vi "4Pi Capture Manager.vi"(7 "Calling VI Ref":refnum<vi>) -> ()   [LabVIEW 2016]
uses:
  4Pi Capture Manager Controls/4Pi Capture Switch Laser.ctl
  4Pi Capture Manager Controls/4Pi Capture Switch Line Scan Modes.ctl
  4Pi Capture Manager Controls/4Pi Capture Line Scan Settings.ctl
  <vilib>/Utility/miscctls.llb/LVPointTypeDef.ctl
  4Pi Capture Manager Controls/4Pi Capture Notifier Type.ctl
  4Pi Capture Manager Controls/4Pi Capture Actions.ctl
  <vilib>/vision/Image Controls.llb/IMAQ Image.ctl
  Hardware Configuration/Hardware Configuration Controls/Device Type.ctl
  Hardware Configuration/Hardware Configuration Controls/Device Function.ctl
  Device Library/Cameras/Hamamatsu/Orca Flash/Orca Flash Controls/Orca Flash Actions.ctl
  Device Library/Cameras/Hamamatsu/Orca Flash/Orca Flash Controls/Orca Flash Parameters.ctl
  Device Library/Cameras/Hamamatsu/Orca Flash/Orca Flash Controls/Orca Flash Parameter List.ctl
  Device Library/Cameras/Hamamatsu/Orca Flash/Orca Flash Controls/Orca Flash ROI.ctl
  4Pi Capture Manager Controls/4Pi Capture Scan Tracker.ctl
  Device Manager/Common Device Queue/Common Device Controls/Common Device Actions.ctl
  Device Library/DAQmx/AO Single Channel Triggered Ramp/AO SCTR Type Defs/AO SCTR Actions.ctl
  Wide Field Drift Correction/WFDC Controls/WFDC External Sync.ctl
  Wide Field Drift Correction/WFDC Controls/WFDC Cycle Pause.ctl
  Wide Field Drift Correction/WFDC Controls/WFDC Status.ctl
  Device Library/Stages/Stages Controls/Stage Actions.ctl
  Device Library/Shutters/Shutter Controls/Shutter Actions.ctl
  Device Library/AOTF and AOM/AOTF Controls/AOTF Actions.ctl
  Device Library/Cameras/Camera Controls/Camera IMAQ Key Info.ctl
  <vilib>/Utility/file.llb/Read Delimited Spreadsheet (DBL).vi
  shell32.dll
panel:
  in  "Main Tab":T1(tab)
  out "Frame":u32(slide) scale=0.0..2.0
  out "Cycle":sgl(slide) scale=0.0..1.0
  in  "Base Save Path":path
  in  "Capture":bool
  in  "Live Preview":bool
  in  "Auto Shutter":bool=TRUE
  out "Z Step":sgl(slide) scale=0.0..1.0
  in  "File Name":string="Test Image"
  in  "Preview Exposure Time (s)":dbl=0.1 caption="Exposure Time (s)"
  in  "Capture Exposure Time (s)":dbl=0.1 caption="Exposure Time (s)"
  in  "No. of Frames":u32=1 min=1
  in  "No. of Cycles":u16=1 min=1
  in  "No. of Z Steps":u16=1 min=1
  in  "Z Step Size (µm)":dbl min=-10.0 max=10.0
  in  "Switch Laser At":T2=enum."Each Cycle"
  out "Current Cycle":u16
  out "Current Step":u16
  out "Current Frame":u32
  in  "Auto Update Subfolder":bool=TRUE
  in  "Subfolder Name":string="Area"
  in  "Current Laser":u16(ring) items=["560", "642"]
  in  "Save As Preset":bool
  in  "Line Scan Active":bool
  in  "Number of Lines":u32=8 min=1 max=200 step=1
  in  "Line Scan Mode":T3
  in  "Line Scanning Presets":u16(ring) items=["01 FPS", "02 FPS", "04 FPS", "08 FPS", "16 FPS", "40 FPS"]
  in  "Line Scan Settings":T4
  in  "Camera Settings":bool
  in  "Quadrants On/Off":bool
  in  "Quit":bool
  # "Live Preview"
  # "Capture"
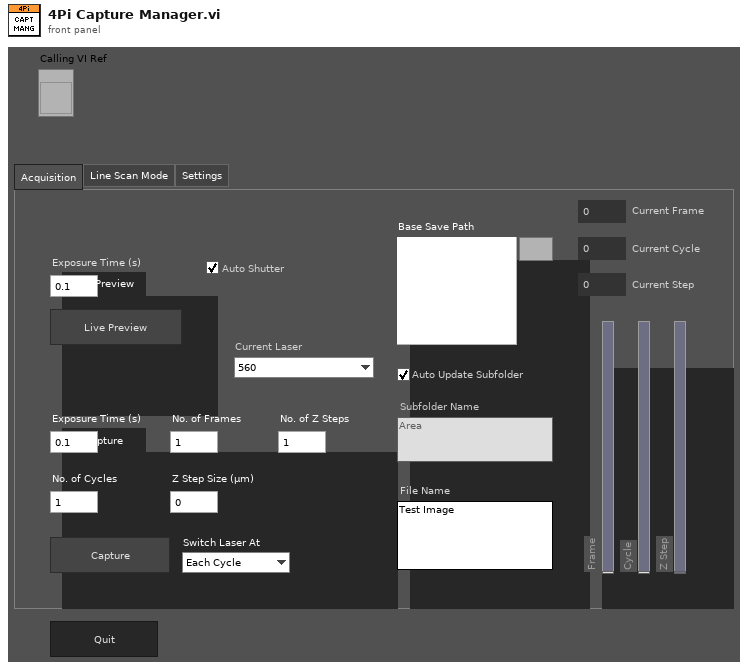
[diagram p1: front panel]
types:
  T1 = enum32{"Acquisition", "Line Scan Mode", "Settings"}
  T2 = typedef "4Pi Capture Switch Laser.ctl" = enum16{"Each Step", "Each Cycle", "All Cycles"}
  T3 = typedef "4Pi Capture Switch Line Scan Modes.ctl" = enum32{"Automatic", "Use Presets", "Manual"}
  T4 = typedef "4Pi Capture Line Scan Settings.ctl" = cluster{"Interline Interval":dbl, "Offset (V)":dbl, "Amplitude (V)":dbl, "Samples Per Channel":dbl, "Delay (ms)":dbl}
  T5 = typedef "IMAQ Image.ctl" = refnum<image>
  T6 = cluster{"Image Ref":T5, "Cycle Number":u16, "Camera Running?":bool, "Capture?":bool}
  T7 = enum8{"Enabled", "Disabled", "Disabled and Grayed Out"}
  T8 = typedef "Device Type.ctl" = enum16{"AOTF", "Camera", "Deformable Mirror", "Laser", "Shutter", "Stage", "Waveform", "Email"}
  T9 = typedef "4Pi Capture Notifier Type.ctl" = cluster{"Actions":T10, "Running?":bool, "Preview Exposure (s)":dbl, "Capture Exposure (s)":dbl, "Cycles":u16, "Frames":u32, "No. of Z Steps":u16, "Z Step Size (µm)":dbl, "Base Path":path, "Init Z Position (µm)":dbl, "Lasers Lines":string[], "Save Path":path, "Line Scan?":bool, "Line Scan Mode":T3, "Metadata File Ref":refnum<file>}
  T10 = typedef "4Pi Capture Actions.ctl" = enum16{"Idle", "Live Preview", "Capture", "Laser On", "Laser Off", "Open Shutters", "Close Shutters", "Set Exposure Time", "Start Acquisition", "Update SubFolder", "Setup", "Camera", "Switch", "Step", "Cycle", "External Cycle Sync", "Write Metadata", "Abort", "Quit"}
  T11 = enum16{"Always On", "Always Off", "Off While Running"}
  T12 = typedef "LVPointTypeDef.ctl" = cluster{"Horizontal":i16, "Vertical":i16}
  T13 = typedef "Image Type" = u32
  T14 = enum32{"Page Enabled", "Page Disabled", "Page Disabled & Grayed"}
  T15 = typedef "Device Function.ctl" = enum16{"Primary", "Secondary", "Overview", "Wide Field Drift Correction", "642 nm Excitation", "560 nm Excitation", "546 nm Excitation", "488 nm Excitation", "405 nm Excitation", "Objective Drift Correction", "4Pi Objective Lock", "Objective XY", "Objective Z", "Sample XY", "Sample Coarse Z", "Sample Z", "4Pi Lower", "4Pi Upper", "Adj Cavity", "Line Scanning", "Alert"}
  T16 = typedef "Orca Flash ROI.ctl" = cluster{"H Offset":i32, "V Offset":i32, "H Width":i32, "V Width":i32}
  T17 = typedef "Orca Flash Parameters.ctl" = cluster{"Value":dbl, "Parameter":T18}
  T18 = typedef "Orca Flash Parameter List.ctl" = u32
  T19 = typedef "Orca Flash Actions.ctl" = enum16{"IDLE", "PREVIEW", "RECORD", "Record Settings", "SETPARAM", "GETPARAM", "SETROI", "GETROI", "PROGRESSIVE MODE", "AREA MODE", "STATUS", "QUIT"}
  T20 = typedef "4Pi Capture Scan Tracker.ctl" = cluster{"Current Step":u16, "Current Cycle":u16, "Current Laser":u16, "# of Lasers":u16, "# of Cycles":u16, "# of Steps":u16, "Switch Laser At":T2}
  T21 = typedef "WFDC Status.ctl" = enum16{"Idle", "Busy", "DC Active", "Error"}
  T22 = typedef "WFDC External Sync.ctl" = cluster{"Cycle Sync":T23, "Z Offset":dbl, "WFDC Status":T21}
  T23 = typedef "WFDC Cycle Pause.ctl" = enum16{"Pause Requested", "Paused", "Resume Requested", "Resumed"}
  T24 = typedef "Stage Actions.ctl" = enum16{"Get Position", "MVR", "MOVE", "HALT", "ONTARGET", "ERROR", "REFERENCE", "INIT", "VELOCITY", "STATUS", "EXIT", "HOME", "ZEROPOS", "NANOPOS", "ANALOG", "QUIT"}
  T25 = typedef "Shutter Actions.ctl" = enum16{"Open", "Close", "Toggle", "Status", "Quit"}
  T26 = typedef "AOTF Actions.ctl" = enum16{"Error Check", "Blank", "Line On/Off", "Set Power", "Status", "Quit"}
  T27 = typedef "AO SCTR Actions.ctl" = enum16{"Stop at Offset", "Update and Run", "Quit"}
  T28 = enum16{"open", "replace", "create", "open or create", "replace or create", "replace or create with confirmation"}
  T29 = typedef "Camera IMAQ Key Info.ctl" = cluster{"Frame":u32, "Sensor Height":i32, "Sensor Width":i32, "ROI Height":i32, "ROI Width":i32, "ROI Enable?":bool, "Bit per Pixel":u8}
  T30 = typedef "Common Device Actions.ctl" = enum16{"Specific Action", "Open Front Panel", "Close Front Panel", "Quit", "Quit All"}
  T31 = typedef "LVRectTypeDef.ctl" = cluster{"Left":i16, "Top":i16, "Right":i16, "Bottom":i16}
  T32 = typedef "LVBoundsTypeDef.ctl" = cluster{"Width":u32, "Height":u32}
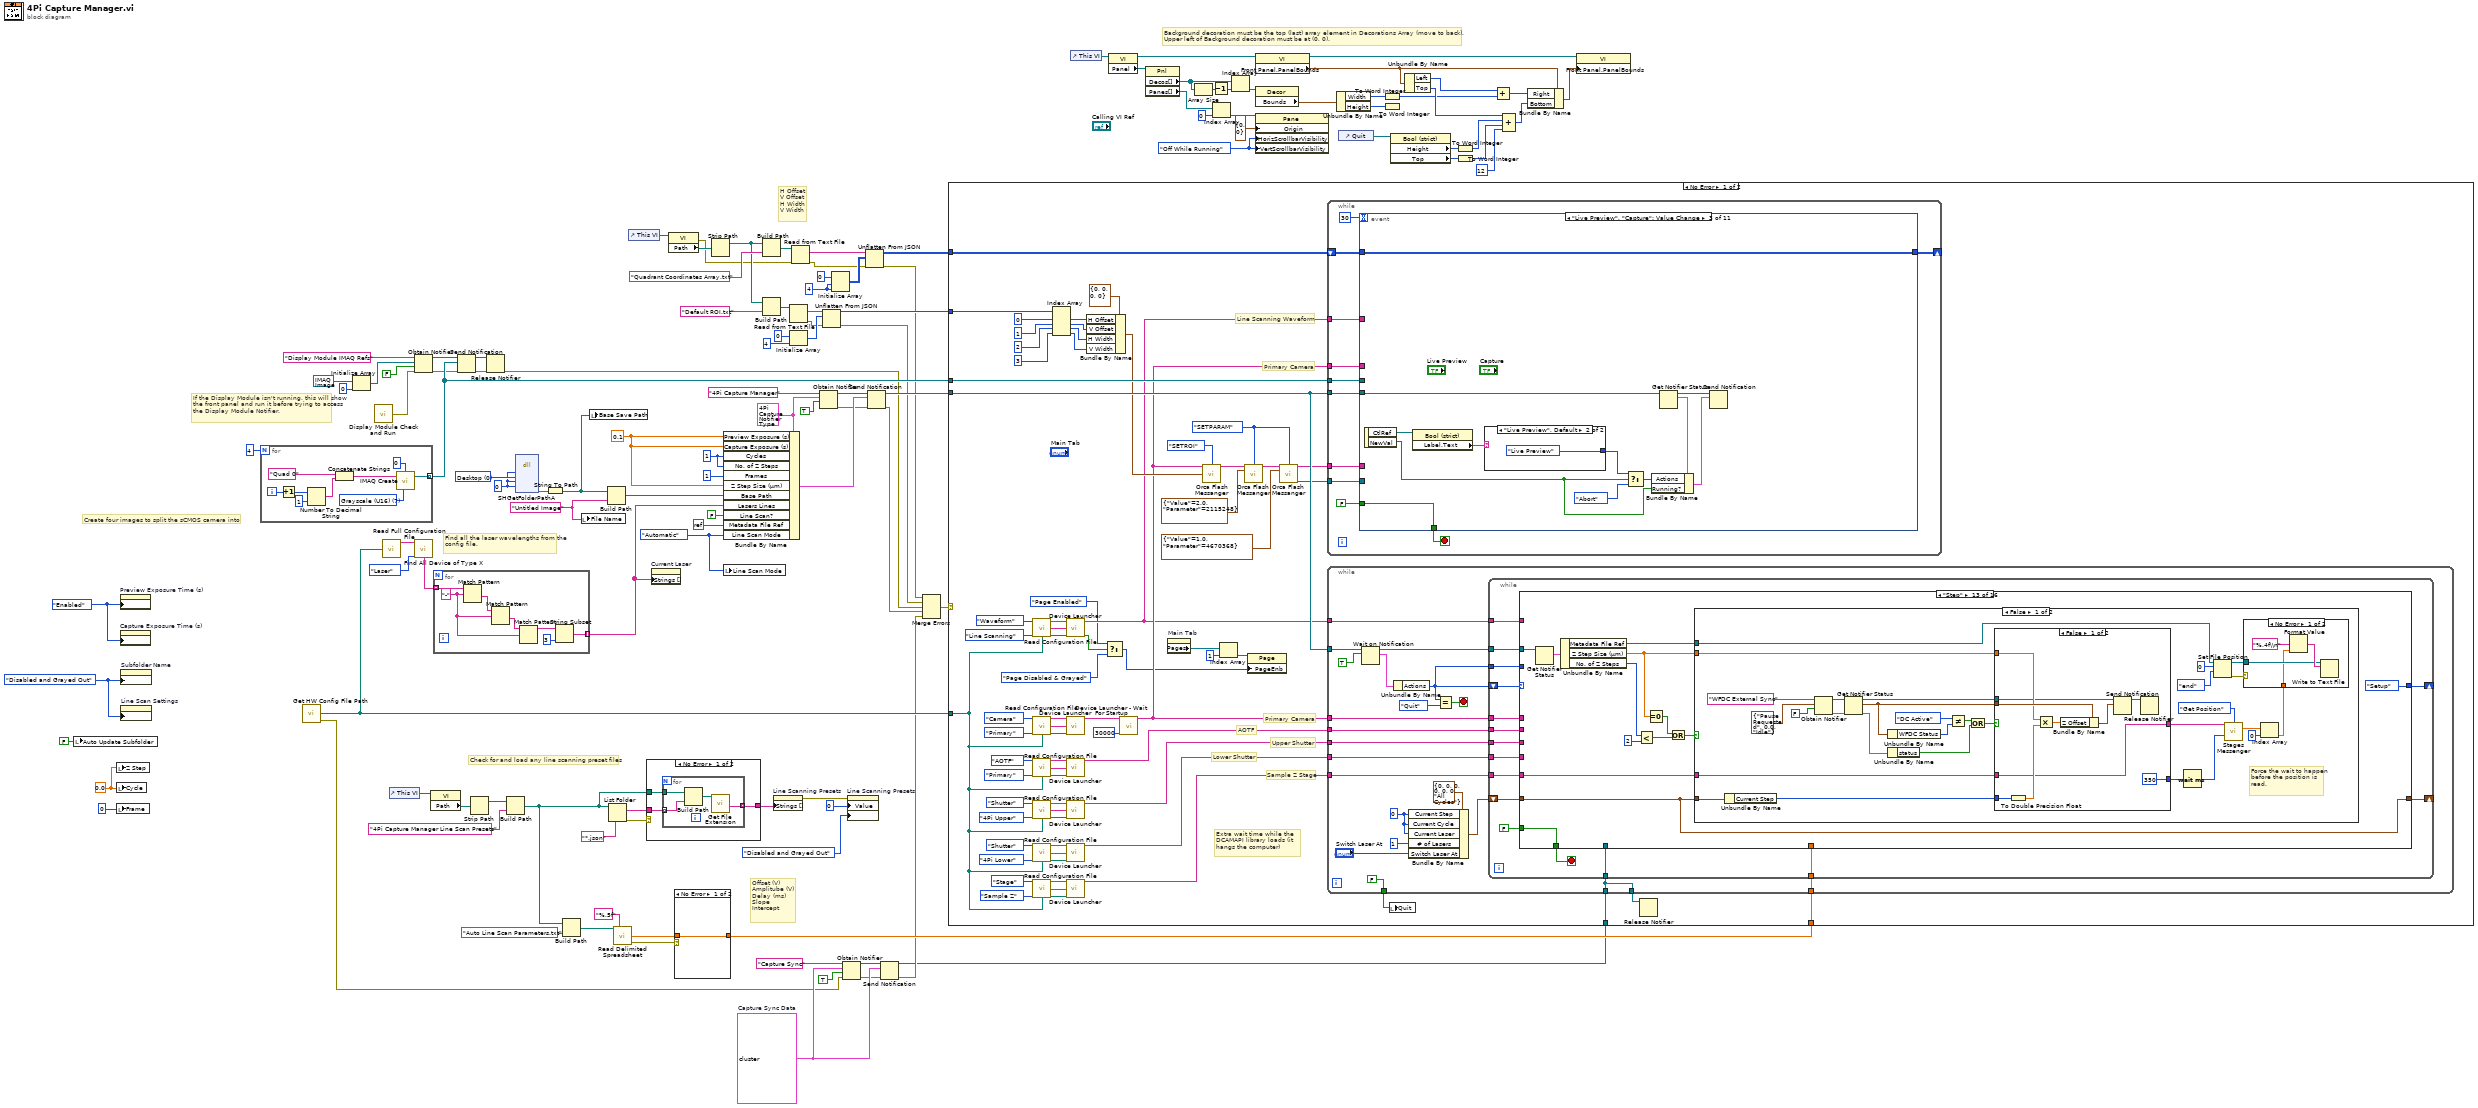
[diagram p0: block diagram]
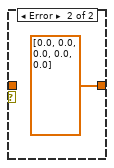
[diagram p2: hidden frame]
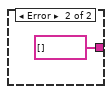
[diagram p3: hidden frame]
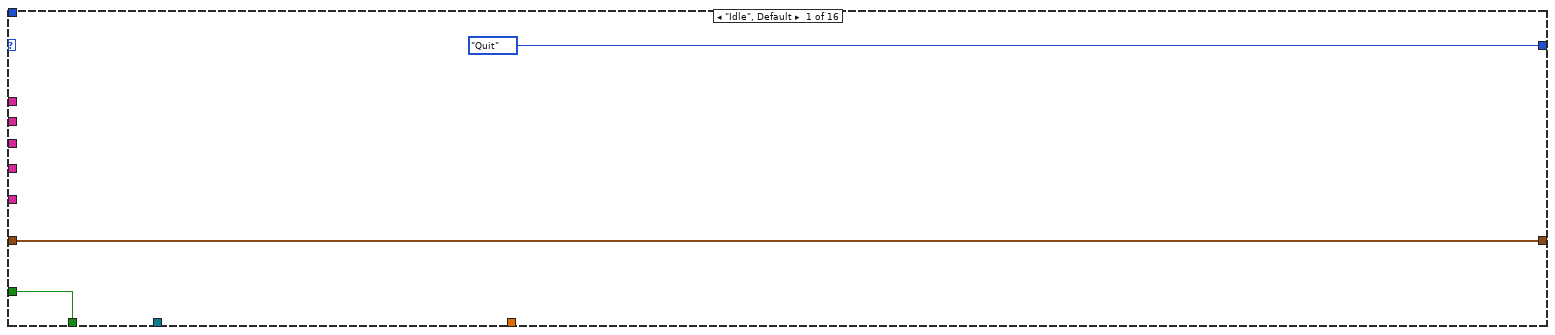
[diagram p4: hidden frame]
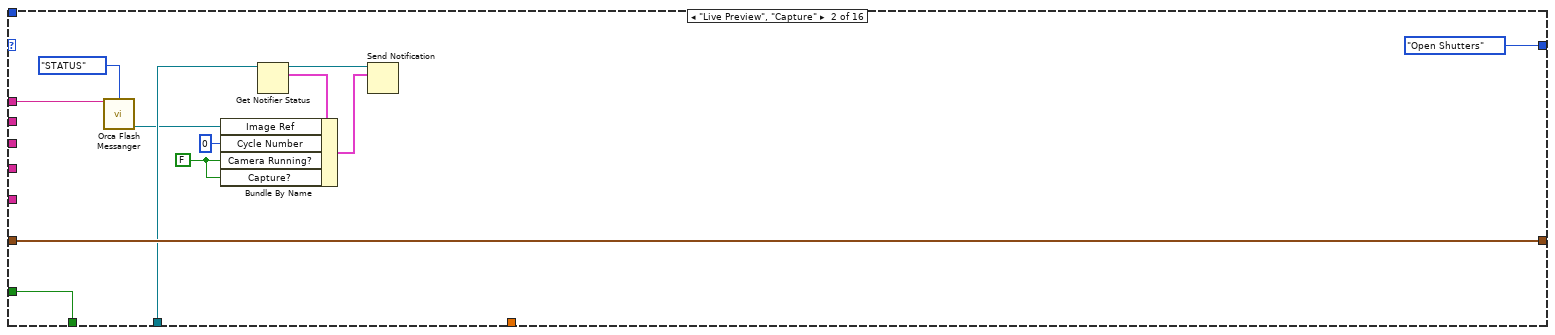
[diagram p5: hidden frame]
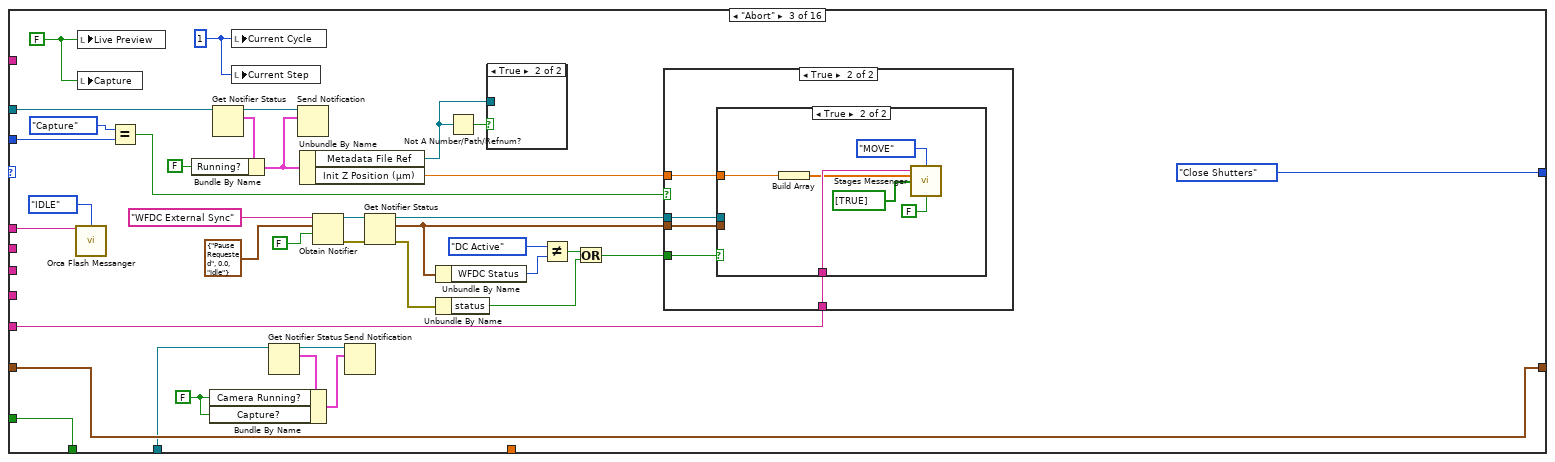
[diagram p6: hidden frame]
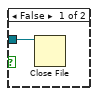
[diagram p7: hidden frame]
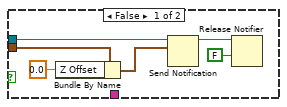
[diagram p9: hidden frame]
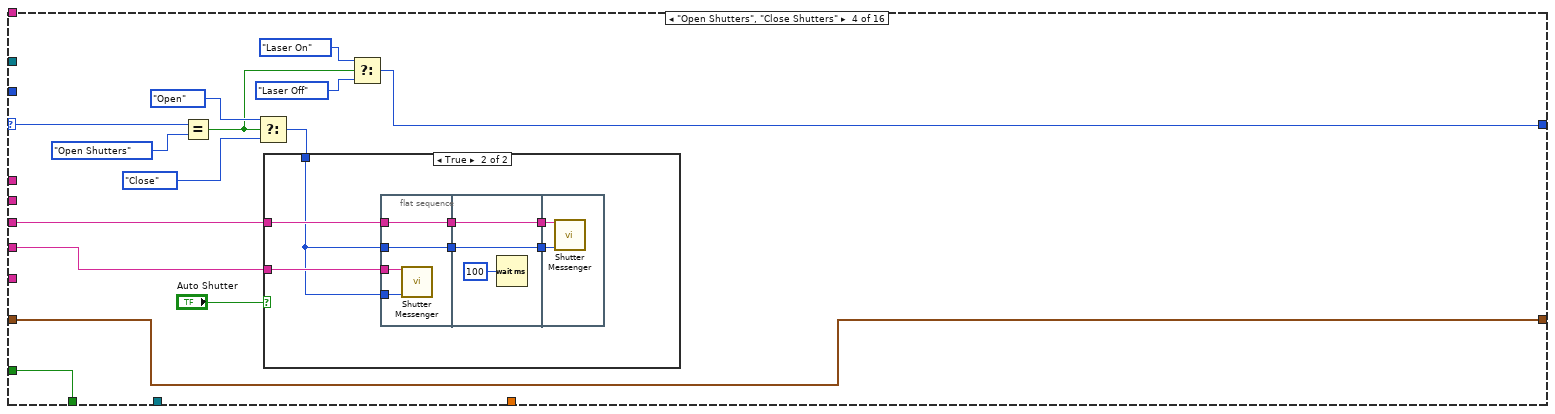
[diagram p10: hidden frame]
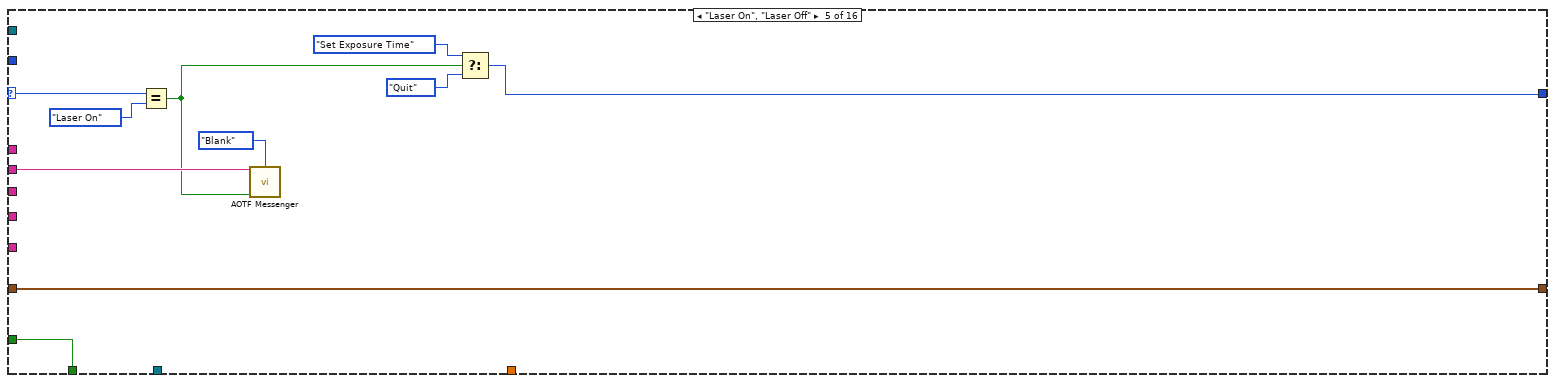
[diagram p12: hidden frame]
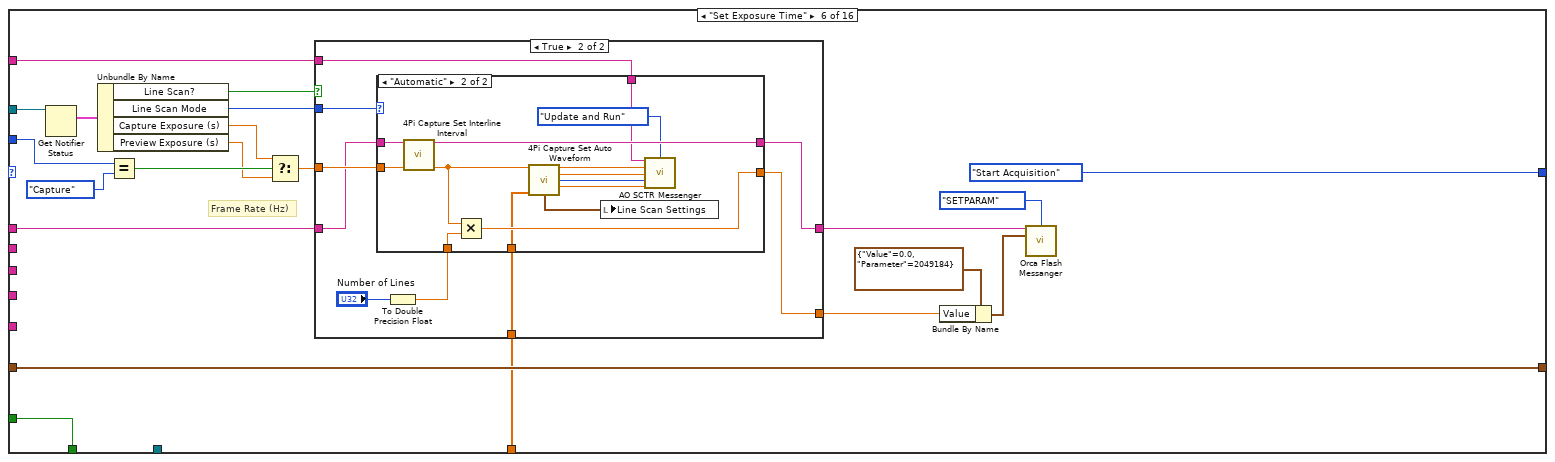
[diagram p13: hidden frame]
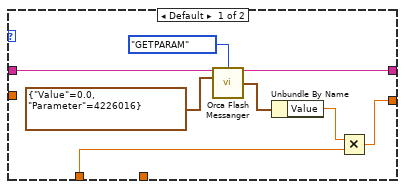
[diagram p15: hidden frame]
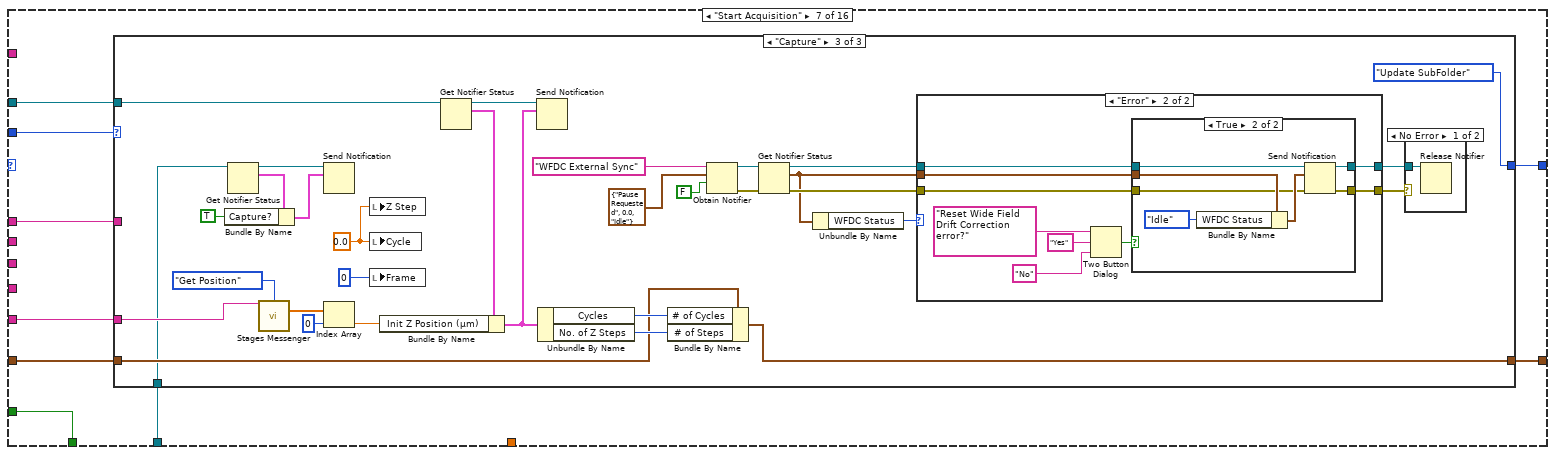
[diagram p16: hidden frame]
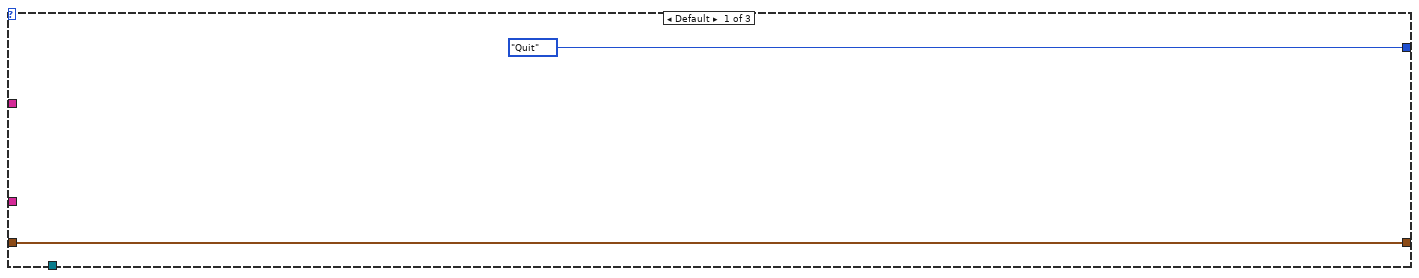
[diagram p17: hidden frame]
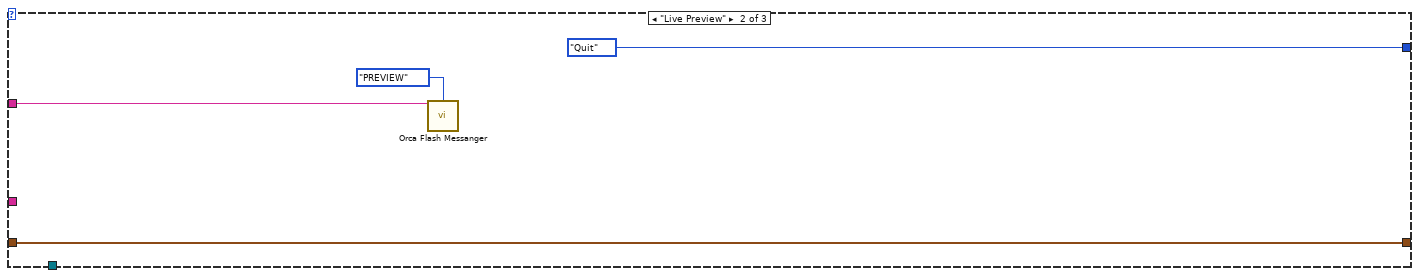
[diagram p18: hidden frame]
diagram:
  w8 = sgl 0.0 ("Cycle")
  w9 = T6 {"Image Ref"=refnum, "Cycle Number"=0, "Camera Running?"=FALSE, "Capture?"=FALSE}  # Capture Sync Data
  w21 = T7."Enabled" ("Disabled")
  w2 = 4Pi_Capture_Switch_Line_Scan_Modes."Automatic" ("Line Scan Mode")
  w22 = T7."Disabled and Grayed Out" ("Disabled")
  w69 = 4 ("dimension size")
  w73 = "Untitled Image"
  w76 = 0 items=["Desktop"=0, "Personal Documents"=5, "AppData"=26, "Local AppData"=28, "Common AppData"=35, "Program Files"=38, "Program Files Common"=43, "Common Documents"=46] ("Requested Path")
  w75 = 0 ("HWND")
  w80 = u16 1 ("Cycles")
  w78 = 0.1 ("Preview Exposure (s)")
  w82 = T9 {"Actions"=enum."Live Preview", "Running?"=FALSE, "Preview Exposure (s)"=0.1, "Capture Exposure (s)"=0.1, "Cycles"=1, "Frames"=0, "No. of Z Steps"=0, "Z Step Size (µm)"=0.0, "Base Path"=path "", "Init Z Position (µm)"=0.0, "Lasers Lines"=[], "Save Path"=path "", "Line Scan?"=FALSE, "Line Scan Mode"=enum."Automatic", "Metadata File Ref"=refnum} ("4Pi Capture Notifier Type")
  w104 = T11."Off While Running" ("Vertical Scrollbar Visibility")
  # "Offset (V)\nAmplitube (V)\nDelay (ms)\nSlope\nIntercept"
  # "Check for and load any line scanning preset files"
  # "Find all the laser wavelengths from the config file."
  # "If the Display Module isn't running, this will show the front panel and run it before trying to access the Display Module Notifier."
  # "H Offset\nV Offset\nH Width\nV Width"
  # "Create four images to split the sCMOS camera into"
  # "Background decoration must be the top (last) array element in Decorations Array (move to back).\nUpper left of Background decoration must be at (0, 0)."
  n1 = local write "Auto Update Subfolder"(FALSE ("Auto Update Subfolder")) -> ()
  n2 = local write "Z Step"(w8) -> ()
  n3 = local write "Cycle"(w8) -> ()
  n4 = local write "Frame"(u32 0 ("Frame")) -> ()
  n5 = property on="Preview Exposure Time (s)" class="DigNum (strict)"("DisabledEnum"=w21) -> ()  [unwired: 2 in, 2 out]
  n6 = property on="Capture Exposure Time (s)" class="DigNum (strict)"("DisabledEnum"=w21) -> ()  [unwired: 2 in, 2 out]
  n7 = property on="Subfolder Name" class="Str"("DisabledEnum"=w22) -> ()  [unwired: 2 in, 2 out]
  n8 = property on="Line Scan Settings" class="Clust (strict)"("DisabledEnum"=w22) -> ()  [unwired: 2 in, 2 out]
  n9 = for {
    N: 4 -> [_]
    tunnel: [w122] -> w86 mode=indexing
    i -> [w130]
    w125 = T13 7 items=["Grayscale (U8)", "Grayscale (I16)", "Grayscale (SGL)", "Complex (CSG)", "RGB (U32)", "HSL (U32)", "RGB (U64)", "Grayscale (U16)"] ("Image Type")
    n10 = Increment(x=w130) -> (x+1=w128:i32)
    n11 = Number To Decimal String(number=w128, width (-)=i16 1) -> (decimal integer string=w126:string)
    n12 = Concatenate Strings("Quad 0" ("name (unnamed)"), w126) -> (w123:string)
    n13 = call "IMAQ Create"("Border Size"=0, "Image Name"=w123, "Image Type"=w125) -> ("New Image"=w122:T5)  [unwired: 2 in, 1 out]
  }
  n14 = call "Get HW Config File Path.vi"() -> ("File Path"=w36:path, "Error"=w6:errorcluster)  [unwired: 14 in]
  n15 = Initialize Array(T5 refnum ("New Image"), 0 ("dimension size")) -> (w41:T5[])
  n16 = call "Display Module Check and Run.vi"() -> ("Error"=w40:errorcluster)  [unwired: 15 in]
  n17 = call "Read Full Configuration File.vi"("Config File Path"=w36) -> ("Unique Notifier Names"=w37:string[])  [unwired: 11 in, 3 out]
  n18 = control-ref of="This VI"() -> (w33:refnum<vi>)
  n19 = Obtain Notifier(name (unnamed)="Display Module IMAQ Refs", notification data type=w41, create if not found? (T)=FALSE, error in (no error)=w40) -> (notifier out=w87:refnum<notifier>, error out=w51:errorcluster)  [unwired: 1 out]
  n20 = call "Find All Device of Type X.vi"("Unique Notifier Names"=w37, "Device Type"=Device_Type."Laser") -> ("All Devices"=w39:string[])  [unwired: 12 in, 1 out]
  n21 = property class="VI"(reference=w33) -> ("Path"=w32:path)  [unwired: 1 in, 2 out]
  n22 = for {
    tunnel: w39 -> [w132] mode=indexing
    tunnel: [w131] -> w13 mode=indexing
    w135 = "-" ("regular expression")
    n23 = Match Pattern(string=w132, regular expression=w135) -> (after substring=w133:string)  [unwired: 1 in, 3 out]
    n24 = Match Pattern(string=w133, regular expression=w135) -> (after substring=w134:string)  [unwired: 1 in, 3 out]
    n25 = Match Pattern(string=w134, regular expression=w135) -> (before substring=w136:string)  [unwired: 1 in, 3 out]
    n26 = String Subset(string=w136, length (rest)=3 ("length (rest)")) -> (substring=w131:string)  [unwired: 1 in]
  }
  n27 = Send Notification(notification=w86, notifier=w87, error in (no error)=w51) -> (notifier out=w71:refnum<notifier>, error out=w56:errorcluster)
  n28 = Strip Path(path=w32) -> (stripped path=w31:path)  [unwired: 1 out]
  n29 = Release Notifier(notifier=w71, error in (no error)=w56) -> (error out=w48:errorcluster)  [unwired: 1 in, 2 out]
  n30 = Build Path(base path=w31, name or relative path="4Pi Capture Manager Line Scan Presets") -> (appended path=w20:path)
  n31 = dll-call lib="shell32.dll" fn="SHGetFolderPathA"("HWND"=w75, "nFolder"=w76, "hToken"=w75, "dwFlags"=w75) -> ("pszPath"=w74:string)  [unwired: 9 in, 2 out]
  n32 = String To Path(string=w74) -> (path=w72:path)
  n33 = Build Path(base path=w20, name or relative path="Auto Line Scan Parameters.txt") -> (appended path=w18:path)
  n34 = local write "File Name"(w73) -> ()
  n35 = local write "Base Save Path"(w72) -> ()
  n36 = Build Path(base path=w72, name or relative path=w73) -> (appended path=w77:path)
  n37 = List Folder(path=w20, pattern="*.json") -> (filenames=w28:string[], error out=w27:errorcluster)  [unwired: 2 in, 2 out]
  n38 = call-poly <vilib>:"Read Delimited Spreadsheet.vi"("file path (dialog if empty)"=w18, "format (%.3f)"="%.5f") -> ("first row"=w15:dbl[], "error out"=w16:errorcluster)  [unwired: 8 in, 4 out]
  n39 = control-ref of="This VI"() -> (w85:refnum<vi>)
  n40 = case shown="No Error" w27 {
    tunnel: w28 -> [w140 _]
    tunnel: w20 -> [w139 _]
    tunnel: [w138 string[] []] -> w26
    frame No Error {
      n41 = for {
        tunnel: w140 -> [w143] mode=indexing
        tunnel: w139 -> [w144]
        tunnel: [w141] -> w138 mode=indexing
        n42 = Build Path(base path=w144, name or relative path=w143) -> (appended path=w142:path)
        n43 = call <vilib>:"Get File Extension.vi"("file"=w142) -> ("filename without extension"=w141:string)  [unwired: 6 in, 4 out]
      }
    }
    frame Error {
    }
  }
  n44 = property on="Current Laser" class="Ring (strict)"("Strings []"=w13) -> ()  [unwired: 2 in, 2 out]
  n45 = property class="VI"(reference=w85) -> (error out=w53:errorcluster, "Path"=w84:path)  [unwired: 1 in, 1 out]
  n46 = case shown="No Error" w16 {
    tunnel: w15 -> [w146 _]
    tunnel: [w146 dbl[] [0.0, 0.0, 0.0, 0.0, 0.0] ("first row")] -> w14
    frame No Error {
    }
    frame Error {
    }
  }
  n47 = Strip Path(path=w84) -> (stripped path=w64:path)  [unwired: 1 out]
  n48 = Bundle By Name(cluster=w82, "Preview Exposure (s)"=w78, "Capture Exposure (s)"=w78, "Cycles"=w80, "No. of Z Steps"=w80, "Frames"=u32 1, "Z Step Size (µm)"=w78, "Base Path"=w77, "Lasers Lines"=w13, "Line Scan?"=FALSE, "Metadata File Ref"=refnum<k0> refnum, "Line Scan Mode"=w2) -> (w81:T9)
  n49 = local write "Line Scan Mode"(w2) -> ()
  n50 = Build Path(base path=w64, name or relative path="Quadrant Coordinates Array.txt") -> (appended path=w67:path)
  n51 = Build Path(base path=w64, name or relative path="Default ROI.txt") -> (appended path=w62:path)
  n52 = property on="Line Scanning Presets" class="Ring (strict)"("Strings []"=w26) -> (error out=w25:errorcluster)  [unwired: 2 in, 1 out]
  n53 = Read from Text File(file (use dialog)=w62) -> (text=w61:string, error out=w54:errorcluster)  [unwired: 3 in, 2 out]
  n54 = Initialize Array(0 ("element"), 4 ("dimension size")) -> (w58:i32[])
  n55 = Read from Text File(file (use dialog)=w67, error in=w53) -> (text=w66:string, error out=w52:errorcluster)  [unwired: 2 in, 2 out]
  n56 = Obtain Notifier(name (unnamed)="4Pi Capture Manager", notification data type=w82, create if not found? (T)=TRUE) -> (notifier out=w90:refnum<notifier>, error out=w55:errorcluster)  [unwired: 1 in, 1 out]
  n57 = Unflatten From JSON(JSON string=w61, type and defaults=w58, error in (no error)=w54) -> (value=w57:i32[], error out=w47:errorcluster)  [unwired: 4 in]
  n58 = Initialize Array(0 ("element"), w69, w69) -> (w68:i32[][])
  n59 = Obtain Notifier(name (unnamed)="Capture Sync", notification data type=w9, create if not found? (T)=TRUE, error in (no error)=w6) -> (notifier out=w10:refnum<notifier>, error out=w5:errorcluster)  [unwired: 1 out]
  n60 = property on="Line Scanning Presets" class="Ring (strict)"(error in=w25, "Value"=u16 0, "DisabledEnum"=T7."Disabled and Grayed Out" ("Disabled")) -> ()  [unwired: 1 in, 2 out]
  n61 = Unflatten From JSON(JSON string=w66, type and defaults=w68, error in (no error)=w52) -> (value=w65:i32[][], error out=w46:errorcluster)  [unwired: 4 in]
  n62 = Send Notification(notification=w81, notifier=w90, error in (no error)=w55) -> (notifier out=w89:refnum<notifier>, error out=w49:errorcluster)
  n63 = Send Notification(notification=w9, notifier=w10, error in (no error)=w5) -> (notifier out=w3:refnum<notifier>, error out=w4:errorcluster)
  n64 = Merge Errors(w46, w47, w48, w49, w4) -> (w50:errorcluster)
  n65 = case shown="No Error" w50 {
    tunnel: w36 -> [w160 _]
    tunnel: w89 -> [w199 w1134]
    tunnel: w86 -> [w187 w1132]
    tunnel: w65 -> [w186 _]
    tunnel: w57 -> [w177 _]
    tunnel: w14 -> [w157 _]
    tunnel: w3 -> [w149 _]
    frame No Error {
      w182 = Orca_Flash_Actions."SETPARAM" ("Camera Actions")
      # "Line Scanning Waveform"
      # "Primary Camera"
      # "Extra wait time while the DCAMAPI library loads (it hangs the computer)"
      # "Sample Z Stage"
      # "Lower Shutter"
      # "Upper Shutter"
      # "AOTF"
      # "Primary Camera"
      n66 = call "Read Configuration File.vi"("Device Type"=Device_Type."Waveform", "Device Function"=Device_Function."Line Scanning", "Config File Path"=w160) -> ("Unique Notifier Name"=w162:string, "Device Ports/IDs/Channels"=w163:string[], "Device Engine Path"=w159:path)  [unwired: 9 in, 1 out]
      n67 = call "Read Configuration File.vi"("Device Type"=Device_Type."Camera", "Device Function"=Device_Function."Primary", "Config File Path"=w160) -> ("Unique Notifier Name"=w219:string, "Device Ports/IDs/Channels"=w218:string[], "Device Engine Path"=w217:path)  [unwired: 9 in, 1 out]
      n68 = call "Read Configuration File.vi"("Device Type"=Device_Type."AOTF", "Device Function"=Device_Function."Primary", "Config File Path"=w160) -> ("Unique Notifier Name"=w210:string, "Device Ports/IDs/Channels"=w211:string[], "Device Engine Path"=w212:path)  [unwired: 9 in, 1 out]
      n69 = call "Read Configuration File.vi"("Device Type"=Device_Type."Shutter", "Device Function"=Device_Function."4Pi Upper", "Config File Path"=w160) -> ("Unique Notifier Name"=w200:string, "Device Ports/IDs/Channels"=w209:string[], "Device Engine Path"=w208:path)  [unwired: 9 in, 1 out]
      n70 = call "Read Configuration File.vi"("Device Type"=Device_Type."Shutter", "Device Function"=Device_Function."4Pi Lower", "Config File Path"=w160) -> ("Unique Notifier Name"=w201:string, "Device Ports/IDs/Channels"=w204:string[], "Device Engine Path"=w205:path)  [unwired: 9 in, 1 out]
      n71 = call "Read Configuration File.vi"("Device Type"=Device_Type."Stage", "Device Function"=Device_Function."Sample Z", "Config File Path"=w160) -> ("Unique Notifier Name"=w194:string, "Device Ports/IDs/Channels"=w192:string[], "Device Engine Path"=w191:path)  [unwired: 9 in, 1 out]
      n72 = Index Array(array=w177, index #1=0 ("index"), index #2=1 ("index"), index #3=2 ("index"), index #4=3 ("index")) -> (element #1=w172:i32, element #2=w169:i32, element #3=w170:i32, element #4=w171:i32)
      n73 = call "Device Launcher.vi"("Notifier Name"=w162, "Device Ports/IDs/Channels"=w163, "Device Engine Path"=w159) -> ("Notifier Name"=w158:string, "Running?"=w153:bool)  [unwired: 11 in]
      n74 = call "Device Launcher.vi"("Notifier Name"=w219, "Device Ports/IDs/Channels"=w218, "Device Engine Path"=w217) -> ("Notifier Name"=w166:string)  [unwired: 11 in, 1 out]
      n75 = call "Device Launcher.vi"("Notifier Name"=w210, "Device Ports/IDs/Channels"=w211, "Device Engine Path"=w212) -> ("Notifier Name"=w198:string)  [unwired: 11 in, 1 out]
      n76 = call "Device Launcher.vi"("Notifier Name"=w200, "Device Ports/IDs/Channels"=w209, "Device Engine Path"=w208) -> ("Notifier Name"=w197:string)  [unwired: 11 in, 1 out]
      n77 = call "Device Launcher.vi"("Notifier Name"=w201, "Device Ports/IDs/Channels"=w204, "Device Engine Path"=w205) -> ("Notifier Name"=w196:string)  [unwired: 11 in, 1 out]
      n78 = call "Device Launcher.vi"("Notifier Name"=w194, "Device Ports/IDs/Channels"=w192, "Device Engine Path"=w191) -> ("Notifier Name"=w189:string)  [unwired: 11 in, 1 out]
      n79 = Bundle By Name(cluster=T16 {"H Offset"=0, "V Offset"=0, "H Width"=0, "V Width"=0} ("Orca Flash ROI"), "H Offset"=w172, "V Offset"=w169, "H Width"=w170, "V Width"=w171) -> (w168:T16)
      n80 = Select(t=T14."Page Enabled" ("Page Enabled State"), s=w153, f=T14."Page Disabled & Grayed" ("Page Enabled State")) -> (s? t:f=w150:T14)
      n81 = call "Device Launcher - Wait For Startup.vi"("Notifier Name"=w166, "Wait Time (ms)"=30000) -> ("Notifier Name (Dup)"=w165:string)  [unwired: 12 in, 1 out]
      n82 = property on="Main Tab" class="TabCtl (strict)"() -> ("Pages"=w156:refnum<vi>[])  [unwired: 2 in, 2 out]
      n83 = call "Orca Flash Messanger.vi"("Notifier Name"=w165, "Camera Actions"=Orca_Flash_Actions."SETROI", "sCMOS ROI"=w168) -> ("Notifier Name Dup"=w185:string)  [unwired: 8 in, 4 out]
      n84 = Index Array(array=w156, index=1) -> (element=w154:refnum<vi>)
      n85 = call "Orca Flash Messanger.vi"("Notifier Name"=w185, "Camera Actions"=w182, "sCMOS Parameter"=T17 {"Value"=2.0, "Parameter"=2115248}) -> ("Notifier Name Dup"=w184:string)  [unwired: 8 in, 4 out]
      n86 = property class="Page"(reference=w154, "PageEnb"=w150) -> ()  [unwired: 1 in, 2 out]
      n87 = call "Orca Flash Messanger.vi"("Notifier Name"=w184, "Camera Actions"=w182, "sCMOS Parameter"=T17 {"Value"=1.0, "Parameter"=4670368}) -> ("Notifier Name Dup"=w183:string, "Image Ref"=w179:T5)  [unwired: 8 in, 3 out]
      n88 = while {
        tunnel: w199 -> [w819]
        tunnel: w183 -> [w818]
        tunnel: w179 -> [w816]
        tunnel: w187 -> [w815]
        shift-right: [w813] -> _
        shift-left: w186 -> [w814]
        tunnel: w165 -> [w812]
        tunnel: w158 -> [w811]
        stop <- w821 stop-if-true
        n89 = event shown="[2] \"Live Preview\", \"Capture\": Value Change" {
          selector: _ -> [_ _ _ _ _ _ _ _ _ _ _]
          dyn-events: _ -> [_ _ _ _ _ _ _ _ _ _ _]
          timeout: 30 -> [_ _ _ _ _ _ _ _ _ _ _]
          tunnel: [w826 w844 w917 w938 w994 w1019 w1041 w1057 w1077 w1101 w1130] -> w821
          tunnel: FALSE -> [w826 w844 w917 w938 w994 w1019 w1041 w1057 w1077 w1101 _]
          tunnel: w819 -> [_ w841 w914 _ _ w1013 w1039 _ w1075 _ w1129]
          tunnel: w818 -> [_ w840 _ _ _ _ _ _ _ _ _]
          tunnel: w816 -> [w824 _ _ w922 _ _ _ _ _ _ _]
          tunnel: w815 -> [w825 _ _ w928 _ _ _ _ _ _ w1117]
          tunnel: w814 -> [w823 w839 w906 w921 w989 w996 w1040 w1058 w1076 w1093 w1116]
          tunnel: [w823 w839 w906 w920 w989 w996 w1040 w1058 w1076 w1093 w1116] -> w813
          tunnel: w812 -> [_ _ _ _ _ w1007 _ _ w1061 _ _]
          tunnel: w811 -> [_ _ _ _ _ w997 _ _ w1069 _ _]
          event Timeout {
            # "Convert to array and then crop. If you\nextract or mask image the destination\nimage custom data keys are overwritten."
            n90 = event-data() -> ()  [unwired: 1 in, 1 out]
            n91 = call "IMAQ ImageToArray"("Image"=w824) -> ("Image Pixels (U16)"=w822:u16[][])  [unwired: 3 in, 4 out]
            n92 = for {
              tunnel: w825 -> [w837] mode=indexing
              tunnel: w822 -> [w838]
              tunnel: w823 -> [w835] mode=indexing
              n93 = Index Array(array=w835, index #1=0 ("index"), index #2=2 ("index"), index #3=1 ("index"), index #4=3 ("index")) -> (element #1=w833:i32, element #2=w832:i32, element #3=w828:i32, element #4=w827:i32)
              n94 = Array Subset(array=w838, index (row)=w833, length (row)=w832, index (col)=w828, length (col)=w827) -> (w836:u16[][])
              n95 = call "IMAQ ArrayToImage"("Image Pixels (U16)"=w836, "Image"=w837) -> ()  [unwired: 8 in, 2 out]
            }
          }
          event "Camera Settings", "Preview Exposure Time (s)", "Capture Exposure Time (s)", "No. of Cycles", "No. of Frames", "No. of Z Steps", "Z Step Size (µm)", "Base Save Path", "File Name": Value Change {
            n96 = event-data() -> ("CtlRef"=w843:refnum<vi>)  [unwired: 1 in]
            n97 = property class="Ctl"(reference=w843) -> ("Label.Text"=w842:string)  [unwired: 1 in, 2 out]
            n98 = case shown="\"Base Save Path\", \"File Name\", \"Save Path\"" w842 {
              tunnel: w841 -> [_ w848 w856 w862 w868 w880 _ w896 w905]
              tunnel: w840 -> [_ _ _ _ _ _ w888 _ _]
              frame Default {
              }
              frame "No. of Cycles" {
                n99 = Get Notifier Status(notifier=w848) -> (notifier out=w847:refnum<notifier>, current notification=w849:T9)  [unwired: 1 in, 3 out]
                n100 = Bundle By Name(cluster=w849, "Cycles"="No. of Cycles", "Actions"=4Pi_Capture_Actions."Idle") -> (w850:T9)
                n101 = Send Notification(notification=w850, notifier=w847) -> ()  [unwired: 1 in, 2 out]
              }
              frame "No. of Frames" {
                n102 = To Double Precision Float(number="No. of Frames") -> (double precision float=w852:dbl)
                n103 = property on="Frame" class="Slide (strict)"("Scale.Maximum"=w852, "Scale.Minimum"=0.0 ("Scale.Range:Minimum")) -> ()  [unwired: 2 in, 2 out]
                n104 = Get Notifier Status(notifier=w856) -> (notifier out=w855:refnum<notifier>, current notification=w857:T9)  [unwired: 1 in, 3 out]
                n105 = Bundle By Name(cluster=w857, "Frames"="No. of Frames", "Actions"=4Pi_Capture_Actions."Idle") -> (w858:T9)
                n106 = Send Notification(notification=w858, notifier=w855) -> ()  [unwired: 1 in, 2 out]
              }
              frame "No. of Z Steps" {
                n107 = Get Notifier Status(notifier=w862) -> (notifier out=w861:refnum<notifier>, current notification=w863:T9)  [unwired: 1 in, 3 out]
                n108 = Bundle By Name(cluster=w863, "No. of Z Steps"="No. of Z Steps", "Actions"=4Pi_Capture_Actions."Idle") -> (w864:T9)
                n109 = Send Notification(notification=w864, notifier=w861) -> ()  [unwired: 1 in, 2 out]
              }
              frame "Z Step Size (µm)" {
                n110 = Get Notifier Status(notifier=w868) -> (notifier out=w867:refnum<notifier>, current notification=w869:T9)  [unwired: 1 in, 3 out]
                n111 = Bundle By Name(cluster=w869, "Z Step Size (µm)"="Z Step Size (µm)", "Actions"=4Pi_Capture_Actions."Idle") -> (w870:T9)
                n112 = Send Notification(notification=w870, notifier=w867) -> ()  [unwired: 1 in, 2 out]
              }
              frame "Base Save Path", "File Name", "Save Path" {
                n113 = Path To String(path="Base Save Path") -> (string=w875:string)
                n114 = Equal?(x="", y=w875) -> (x = y?=w873:bool)
                n115 = case shown="False" w873 {
                  tunnel: [w883 w884] -> w872
                  tunnel: "Base Save Path" -> [w883 _]
                  frame False {
                  }
                  frame True {
                    w887 = 0 items=["Desktop"=0, "Personal Documents"=5, "AppData"=26, "Local AppData"=28, "Common AppData"=35, "Program Files"=38, "Program Files Common"=43, "Common Documents"=46] ("Requested Path")
                    w886 = 0 ("HWND")
                    n116 = dll-call lib="shell32.dll" fn="SHGetFolderPathA"("HWND"=w886, "nFolder"=w887, "hToken"=w886, "dwFlags"=w886) -> ("pszPath"=w885:string)  [unwired: 9 in, 2 out]
                    n117 = String To Path(string=w885) -> (path=w884:path)
                  }
                }
                n118 = Build Path(base path=w872, name or relative path="File Name") -> (appended path=w876:path)
                n119 = Get Notifier Status(notifier=w880) -> (notifier out=w879:refnum<notifier>, current notification=w881:T9)  [unwired: 1 in, 3 out]
                n120 = Bundle By Name(cluster=w881, "Base Path"=w876, "Actions"=4Pi_Capture_Actions."Idle") -> (w882:T9)
                n121 = Send Notification(notification=w882, notifier=w879) -> ()  [unwired: 1 in, 2 out]
              }
              frame "Camera Settings" {
                n122 = Select(t=Common_Device_Actions."Open Front Panel" ("Common Actions"), s="Camera Settings", f=Common_Device_Actions."Close Front Panel" ("Common Actions")) -> (s? t:f=w892:T30)
                n123 = call "Common Device Queue Messenger.vi"("Common Action"=w892, "Notifier Name"=w888) -> ()  [unwired: 13 in, 1 out]
              }
              frame "Preview Exposure Time (s)" {
                # "Add in a preview stop\nand restart here"
                n124 = Get Notifier Status(notifier=w896) -> (notifier out=w899:refnum<notifier>, current notification=w898:T9)  [unwired: 1 in, 3 out]
                n125 = Bundle By Name(cluster=w898, "Preview Exposure (s)"="Preview Exposure Time (s)", "Running?"=FALSE ("Abort"), "Actions"=4Pi_Capture_Actions."Idle") -> (w897:T9)
                n126 = Send Notification(notification=w897, notifier=w899) -> ()  [unwired: 1 in, 2 out]
              }
              frame "Capture Exposure Time (s)" {
                n127 = Get Notifier Status(notifier=w905) -> (notifier out=w904:refnum<notifier>, current notification=w903:T9)  [unwired: 1 in, 3 out]
                n128 = Bundle By Name(cluster=w903, "Capture Exposure (s)"="Capture Exposure Time (s)", "Actions"=4Pi_Capture_Actions."Idle") -> (w902:T9)
                n129 = Send Notification(notification=w902, notifier=w904) -> ()  [unwired: 1 in, 2 out]
              }
            }
          }
          event "Live Preview", "Capture": Value Change {
            n130 = event-data() -> ("CtlRef"=w909:refnum<vi>, "NewVal"=w912:bool)  [unwired: 1 in]
            n131 = property class="Bool (strict)"(reference=w909) -> ("Label.Text"=w908:string)  [unwired: 1 in, 2 out]
            n132 = case shown="\"Live Preview\", Default" w908 {
              tunnel: [4Pi_Capture_Actions."Capture" ("y") 4Pi_Capture_Actions."Live Preview" ("y")] -> w907
              frame "Capture" {
              }
              frame "Live Preview", Default {
              }
            }
            n133 = Select(t=w907, s=w912, f=4Pi_Capture_Actions."Abort" ("y")) -> (s? t:f=w911:T10)
            n134 = Get Notifier Status(notifier=w914) -> (notifier out=w915:refnum<notifier>, current notification=w913:T9)  [unwired: 1 in, 3 out]
            n135 = Bundle By Name(cluster=w913, "Actions"=w911, "Running?"=w912) -> (w910:T9)
            n136 = Send Notification(notification=w910, notifier=w915) -> ()  [unwired: 1 in, 2 out]
          }
          event "Quadrants On/Off": Value Change {
            n137 = event-data() -> ("NewVal"=w934:bool)  [unwired: 1 in]
            n138 = Obtain Notifier(name (unnamed)="Display Module IMAQ Refs", notification data type=T5[] [], create if not found? (T)=FALSE) -> (notifier out=w927:refnum<notifier>, error out=w926:errorcluster)  [unwired: 1 in, 1 out]
            n139 = Get Notifier Status(notifier=w927, error in (no error)=w926) -> (notifier out=w925:refnum<notifier>, current notification=w923:T5[], error out=w924:errorcluster)  [unwired: 2 out]
            n140 = case shown="False" w934 {
              tunnel: w925 -> [w960 w975]
              tunnel: w924 -> [w959 w974]
              tunnel: [w956 w970] -> w930
              tunnel: [w960 w975] -> w931
              tunnel: [w959 w974] -> w929
              tunnel: w928 -> [w951 w973]
              tunnel: w923 -> [w958 w972]
              tunnel: w922 -> [w952 w969]
              tunnel: w921 -> [_ w968]
              tunnel: [w939 w968] -> w920
              frame False {
                w950 = 4 ("dimension size")
                n141 = control-ref of="This VI"() -> (w940:refnum<vi>)
                n142 = Equal?(x=w958, y=w952) -> (x = y?=w955:bool[])
                n143 = property class="VI"(reference=w940) -> (error out=w948:errorcluster, "Path"=w941:path)  [unwired: 1 in, 1 out]
                n144 = for {
                  tunnel: w955 -> [w967] mode=indexing
                  tunnel: [w966] -> w953
                  i -> [w966]
                  stop <- w967 stop-if-true
                }
                n145 = Or Array Elements(Boolean array=w955) -> (logical OR=w954:bool)
                n146 = Strip Path(path=w941) -> (stripped path=w947:path)  [unwired: 1 out]
                n147 = case shown="True" w954 {
                  tunnel: w953 -> [_ w964]
                  tunnel: w958 -> [w961 w963]
                  tunnel: [w961 w962] -> w957
                  frame False {
                  }
                  frame True {
                    n148 = Delete From Array(array=w963, length=1, index=w964) -> (array with subset deleted=w962:T5[])  [unwired: 1 out]
                  }
                }
                n149 = Build Path(base path=w947, name or relative path="Quadrant Coordinates Array.txt") -> (appended path=w945:path)
                n150 = Read from Text File(file (use dialog)=w945, error in=w948) -> (text=w946:string, error out=w949:errorcluster)  [unwired: 2 in, 2 out]
                n151 = Initialize Array(0 ("element"), w950, w950) -> (w944:i32[][])
                n152 = Build Array (concatenate)(w957, w951) -> (w956:T5[])
                n153 = Unflatten From JSON(JSON string=w946, type and defaults=w944, error in (no error)=w949) -> (value=w939:i32[][])  [unwired: 4 in, 1 out]
              }
              frame True {
                n154 = for {
                  tunnel: w973 -> [w978] mode=indexing
                  shift-right: [w976] -> w971
                  shift-left: w972 -> [w977]
                  n155 = Equal?(x=w977, y=w978) -> (x = y?=w981:bool[])
                  n156 = for {
                    tunnel: w981 -> [w988] mode=indexing
                    tunnel: [w987] -> w979
                    i -> [w987]
                    stop <- w988 stop-if-true
                  }
                  n157 = Or Array Elements(Boolean array=w981) -> (logical OR=w980:bool)
                  n158 = case shown="True" w980 {
                    tunnel: w979 -> [_ w985]
                    tunnel: w977 -> [w982 w984]
                    tunnel: [w982 w983] -> w976
                    frame False {
                    }
                    frame True {
                      n159 = Delete From Array(array=w984, length=1, index=w985) -> (array with subset deleted=w983:T5[])  [unwired: 1 out]
                    }
                  }
                }
                n160 = Build Array (concatenate)(w971, w969) -> (w970:T5[])
              }
            }
            n161 = Send Notification(notification=w930, notifier=w931, error in (no error)=w929) -> (notifier out=w933:refnum<notifier>, error out=w932:errorcluster)
            n162 = Release Notifier(notifier=w933, error in (no error)=w932) -> ()  [unwired: 1 in, 3 out]
          }
          event "Auto Update Subfolder": Value Change {
            n163 = event-data() -> ("NewVal"=w993:bool)  [unwired: 1 in]
            n164 = Select(t=T7."Enabled" ("Disabled"), s=w993, f=T7."Disabled and Grayed Out") -> (s? t:f=w990:T7)
            n165 = property on="Subfolder Name" class="Str"("DisabledEnum"=w990) -> ()  [unwired: 2 in, 2 out]
          }
          event "Line Scan Active": Value Change {
            n166 = event-data() -> ("NewVal"=w995:bool)  [unwired: 1 in]
            n167 = Select(t="Frame Rate (Hz)", s=w995, f="Exposure Time (s)") -> (s? t:f=w1016:string)
            n168 = Select(t=4.0, s=w995, f=0.1) -> (s? t:f=w1009:dbl)
            n169 = Select(t=-1.0 ("f"), s=w995, f=0.0) -> (s? t:f=w1000:dbl)
            n170 = Select(t=AO_SCTR_Actions."Update and Run" ("Actions"), s=w995, f=AO_SCTR_Actions."Stop at Offset" ("Actions")) -> (s? t:f=w1001:T27)
            n171 = property on="Capture Exposure Time (s)" class="DigNum (strict)"("Caption.Text"=w1016, "Value"=w1009) -> ()  [unwired: 2 in, 2 out]
            n172 = property on="Preview Exposure Time (s)" class="DigNum (strict)"("Caption.Text"=w1016, "Value"=w1009) -> ()  [unwired: 2 in, 2 out]
            n173 = call "AO SCTR Messenger.vi"("Notifier Name"=w997, "Actions"=w1001, "Offset (V)"=w1000) -> ()  [unwired: 12 in, 1 out]
            n174 = case shown="False" w995 {
              frame False {
                w1020 = T7."Enabled" ("Disabled")
                n175 = property on="Preview Exposure Time (s)" class="DigNum (strict)"("DisabledEnum"=w1020) -> ()  [unwired: 2 in, 2 out]
                n176 = property on="Capture Exposure Time (s)" class="DigNum (strict)"("DisabledEnum"=w1020) -> ()  [unwired: 2 in, 2 out]
              }
              frame True {
              }
            }
            n177 = Get Notifier Status(notifier=w1013) -> (notifier out=w1012:refnum<notifier>, current notification=w1011:T9)  [unwired: 1 in, 3 out]
            n178 = Bundle By Name(cluster=w1011, "Line Scan?"=w995, "Actions"=4Pi_Capture_Actions."Idle", "Preview Exposure (s)"=w1009, "Capture Exposure (s)"=w1009) -> (w1008:T9)
            n179 = Select(t=Orca_Flash_Actions."PROGRESSIVE MODE" ("Camera Actions"), s=w995, f=Orca_Flash_Actions."AREA MODE" ("Camera Actions")) -> (s? t:f=w1004:T19)
            n180 = call "Orca Flash Messanger.vi"("Notifier Name"=w1007, "Camera Actions"=w1004) -> ()  [unwired: 9 in, 5 out]
            n181 = Send Notification(notification=w1008, notifier=w1012) -> ()  [unwired: 1 in, 2 out]
          }
          event Value Change {
            n182 = event-data() -> ("NewVal"=w1030:T3)  [unwired: 1 in]
            n183 = Get Notifier Status(notifier=w1039) -> (notifier out=w1038:refnum<notifier>, current notification=w1037:T9)  [unwired: 1 in, 3 out]
            n184 = Bundle By Name(cluster=w1037, "Actions"=4Pi_Capture_Actions."Idle", "Line Scan Mode"=w1030) -> (w1036:T9)
            n185 = Send Notification(notification=w1036, notifier=w1038) -> ()  [unwired: 1 in, 2 out]
            n186 = Equal?(x=w1030, y=4Pi_Capture_Switch_Line_Scan_Modes."Use Presets") -> (x = y?=w1022:bool)
            n187 = Not Equal?(x=w1030, y=4Pi_Capture_Switch_Line_Scan_Modes."Automatic") -> (x != y?=w1024:bool)
            n188 = Select(t=T7."Enabled" ("Disabled"), s=w1022, f=T7."Disabled and Grayed Out" ("Disabled")) -> (s? t:f=w1032:T7)
            n189 = property on="Line Scanning Presets" class="Ring (strict)"("DisabledEnum"=w1032) -> ()  [unwired: 2 in, 2 out]
            n190 = case shown="True" w1022 {
              frame False {
              }
              frame True {
                n191 = property on="Line Scanning Presets" class="Ring (strict)"() -> ("Value"=w1042:u16)  [unwired: 2 in, 2 out]
                n192 = property on="Line Scanning Presets" class="Ring (strict)"("Val(Sgnl)"=w1042) -> ()  [unwired: 2 in, 2 out]
              }
            }
            n193 = Select(t=T7."Disabled and Grayed Out" ("Disabled"), s=w1024, f=T7."Enabled" ("Disabled")) -> (s? t:f=w1023:T7)
            n194 = Select(t=T7."Enabled" ("Disabled"), s=w1024, f=T7."Disabled and Grayed Out" ("Disabled")) -> (s? t:f=w1027:T7)
            n195 = property on="Preview Exposure Time (s)" class="DigNum (strict)"("DisabledEnum"=w1023) -> ()  [unwired: 2 in, 2 out]
            n196 = property on="Capture Exposure Time (s)" class="DigNum (strict)"("DisabledEnum"=w1023) -> ()  [unwired: 2 in, 2 out]
            n197 = property on="Save As Preset" class="Bool"("DisabledEnum"=w1027) -> ()  [unwired: 2 in, 2 out]
            n198 = property on="Line Scan Settings" class="Clust (strict)"("DisabledEnum"=w1027) -> ()  [unwired: 2 in, 2 out]
          }
          event "Line Scanning Presets": Value Change {
            n199 = event-data() -> ("CtlRef"=w1052:refnum<vi>)  [unwired: 1 in]
            n200 = control-ref of="This VI"() -> (w1056:refnum<vi>)
            n201 = property class="Ring (strict)"(reference=w1052) -> ("RingText.Text"=w1050:string)  [unwired: 1 in, 2 out]
            n202 = property class="VI"(reference=w1056) -> ("Path"=w1055:path)  [unwired: 1 in, 2 out]
            n203 = Strip Path(path=w1055) -> (stripped path=w1054:path)  [unwired: 1 out]
            n204 = Concatenate Strings(w1050, ".json" ("string")) -> (w1048:string)
            n205 = Build Path(base path=w1054, name or relative path="4Pi Capture Manager Line Scan Presets") -> (appended path=w1051:path)
            n206 = Build Path(base path=w1051, name or relative path=w1048) -> (appended path=w1047:path)
            n207 = Read from Text File(file (use dialog)=w1047) -> (text=w1046:string, error out=w1044:errorcluster)  [unwired: 3 in, 2 out]
            n208 = Unflatten From JSON(JSON string=w1046, type and defaults=T4 {"Interline Interval"=0.0, "Offset (V)"=0.0, "Amplitude (V)"=0.0, "Samples Per Channel"=0.0, "Delay (ms)"=0.0} ("Line Scan Settings"), error in (no error)=w1044) -> (value=w1043:T4)  [unwired: 4 in, 1 out]
            n209 = property on="Line Scan Settings" class="Clust (strict)"("Val(Sgnl)"=w1043) -> ()  [unwired: 2 in, 2 out]
          }
          event Value Change {
            # "If you try and set the ILI while the camera is in area mode it gives an error"
            n210 = event-data() -> ("NewVal"=w1070:T4)  [unwired: 1 in]
            n211 = Get Notifier Status(notifier=w1075) -> (current notification=w1074:T9)  [unwired: 1 in, 4 out]
            n212 = Unbundle By Name(w1070) -> ("Offset (V)"=w1064:dbl, "Amplitude (V)"=w1068:dbl, "Samples Per Channel"=w1067:dbl, "Delay (ms)"=w1066:dbl, "Interline Interval"=w1060:dbl)
            n213 = Unbundle By Name(w1074) -> ("Line Scan?"=w1059:bool)
            n214 = To Long Integer(number=w1067) -> (32bit integer=w1065:i32)
            n215 = Select(t=w1064, s=w1059, f=0.0) -> (s? t:f=w1062:dbl)
            n216 = Select(t=AO_SCTR_Actions."Update and Run" ("Actions"), s=w1059, f=AO_SCTR_Actions."Stop at Offset" ("Actions")) -> (s? t:f=w1071:T27)
            n217 = call "AO SCTR Messenger.vi"("Notifier Name"=w1069, "Actions"=w1071, "Offset (V)"=w1062, "Amplitude (V)"=w1068, "Samples Per Channel"=w1065, "Start Delay (ms)"=w1066) -> ()  [unwired: 9 in, 1 out]
            n218 = case shown="True" w1059 {
              tunnel: w1061 -> [_ w1080]
              tunnel: w1060 -> [_ w1079]
              frame False {
              }
              frame True {
                n219 = Bundle By Name(cluster=T17 {"Value"=0.0, "Parameter"=4226016} ("sCMOS Parameter"), "Value"=w1079) -> (w1083:T17)
                n220 = call "Orca Flash Messanger.vi"("Notifier Name"=w1080, "Camera Actions"=Orca_Flash_Actions."SETPARAM", "sCMOS Parameter"=w1083) -> ("sCMOS Parameter"=w1084:T17)  [unwired: 8 in, 4 out]
                n221 = Unbundle By Name(w1084) -> ("Value"=w1078:dbl)
                n222 = property on="Interline Interval" class="DigNum (strict)"("Value"=w1078) -> ()  [unwired: 2 in, 2 out]
              }
            }
          }
          event "Save As Preset": Value Change {
            n223 = event-data() -> ()  [unwired: 1 in, 6 out]
            n224 = control-ref of="This VI"() -> (w1097:refnum<vi>)
            n225 = property class="VI"(reference=w1097) -> ("Path"=w1096:path)  [unwired: 1 in, 2 out]
            n226 = Strip Path(path=w1096) -> (stripped path=w1095:path)  [unwired: 1 out]
            n227 = Build Path(base path=w1095, name or relative path="4Pi Capture Manager Line Scan Presets") -> (appended path=w1086:path)
            n228 = call "File Dialog"("start path"=w1086, "prompt"="Save Preset File", "pattern (all files)"="*.json", "pattern label"="JSON") -> ("selected path"=w1091:path, "error out"=w1092:errorcluster)  [unwired: 8 in, 2 out]
            n229 = case shown="Error" w1092 {
              selector: w1092 -> [_ w1115]
              tunnel: w1091 -> [w1114 _]
              tunnel: [w1110 w1115] -> w1085
              frame No Error {
                n230 = local read "Line Scan Settings"() -> (w1113:T4)
                n231 = Flatten To JSON(anything=w1113) -> (JSON string=w1112:string, 11:w1111:errorcluster)  [unwired: 2 in]
                n232 = Write to Text File(file (use dialog)=w1114, text=w1112, error in=w1111) -> (error out=w1110:errorcluster)  [unwired: 1 in, 2 out]
              }
              frame Error {
              }
            }
            n233 = List Folder(path=w1086, pattern="*.json", error in=w1085) -> (filenames=w1089:string[], error out=w1088:errorcluster)  [unwired: 1 in, 2 out]
            n234 = case shown="No Error" w1088 {
              tunnel: w1089 -> [w1104 _]
              tunnel: w1086 -> [w1103 _]
              tunnel: [w1102 string[] []] -> w1087
              frame No Error {
                n235 = for {
                  tunnel: w1104 -> [w1107] mode=indexing
                  tunnel: w1103 -> [w1108]
                  tunnel: [w1105] -> w1102 mode=indexing
                  n236 = Build Path(base path=w1108, name or relative path=w1107) -> (appended path=w1106:path)
                  n237 = call <vilib>:"Get File Extension.vi"("file"=w1106) -> ("filename without extension"=w1105:string)  [unwired: 6 in, 4 out]
                }
              }
              frame Error {
              }
            }
            n238 = property on="Line Scanning Presets" class="Ring (strict)"("Strings []"=w1087) -> ()  [unwired: 2 in, 2 out]
          }
          event "Quit": Value Change {
            n239 = event-data() -> ("NewVal"=w1130:bool)  [unwired: 1 in]
            n240 = Get Notifier Status(notifier=w1129) -> (notifier out=w1128:refnum<notifier>, current notification=w1127:T9)  [unwired: 1 in, 3 out]
            n241 = Bundle By Name(cluster=w1127, "Running?"=FALSE ("Abort"), "Actions"=4Pi_Capture_Actions."Quit") -> (w1121:T9)
            n242 = Send Notification(notification=w1121, notifier=w1128) -> (notifier out=w1125:refnum<notifier>)  [unwired: 1 in, 1 out]
            n243 = Wait on Notification(notifier=w1125, ignore previous (F)=TRUE, timeout in ms (-1)=500) -> (notifier out=w1122:refnum<notifier>)  [unwired: 1 in, 3 out]
            n244 = Send Notification(notification=w1121, notifier=w1122) -> (notifier out=w1119:refnum<notifier>)  [unwired: 1 in, 1 out]
            n245 = Release Notifier(notifier=w1119, force destroy? (F)=TRUE) -> ()  [unwired: 1 in, 3 out]
            n246 = for {
              tunnel: w1117 -> [w1131] mode=indexing
              n247 = call "IMAQ Dispose"("Image"=w1131) -> ()  [unwired: 5 in, 1 out]
            }
          }
        }
      }
      n248 = while {
        tunnel: w199 -> [w240]
        tunnel: w165 -> [w234]
        tunnel: w198 -> [w232]
        tunnel: w197 -> [w231]
        tunnel: w196 -> [w230]
        tunnel: [FALSE] -> w195
        tunnel: w189 -> [w228]
        tunnel: w158 -> [w222]
        tunnel: w157 -> [w221]
        tunnel: w149 -> [w220]
        tunnel: [w220] -> w148
        stop <- w236 stop-if-true
        w226 = u16 0 ("Current Step")
        n249 = Wait on Notification(notifier=w240, ignore previous (F)=TRUE) -> (notifier out=w235:refnum<notifier>, notification=w238:T9)  [unwired: 2 in, 2 out]
        n250 = Unbundle By Name(w238) -> ("Actions"=w233:T10)
        n251 = Bundle By Name(cluster=T20 {"Current Step"=0, "Current Cycle"=0, "Current Laser"=0, "# of Lasers"=0, "# of Cycles"=0, "# of Steps"=0, "Switch Laser At"=enum."All Cycles"} ("Cluster"), "Current Step"=w226, "Current Cycle"=w226, "Current Laser"=w226, "# of Lasers"=u16 1, "Switch Laser At"="Switch Laser At") -> (w224:T20)
        n252 = Equal?(x=w233, y=4Pi_Capture_Actions."Quit") -> (x = y?=w236:bool)
        n253 = while {
          shift-right: [w255] -> _
          shift-left: w233 -> [w256]
          tunnel: w235 -> [w247]
          tunnel: w234 -> [w252]
          tunnel: w233 -> [w251]
          tunnel: w232 -> [w250]
          tunnel: w231 -> [w249]
          tunnel: w230 -> [w248]
          tunnel: w228 -> [w246]
          shift-right: [w244] -> _
          shift-left: w224 -> [w245]
          tunnel: w222 -> [w243]
          tunnel: w221 -> [w242]
          tunnel: w220 -> [w241]
          stop <- w253 stop-if-true
          n254 = case shown="\"Step\"" w256 {
            selector: w256 -> [_ _ _ w338 w366 _ _ _ _ _ _ _ _ _ _ _]
            tunnel: [4Pi_Capture_Actions."Quit" ("y") 4Pi_Capture_Actions."Open Shutters" ("y") 4Pi_Capture_Actions."Close Shutters" ("y") w329 w360 4Pi_Capture_Actions."Start Acquisition" ("y") w427 4Pi_Capture_Actions."Write Metadata" ("y") 4Pi_Capture_Actions."Setup" ("y") 4Pi_Capture_Actions."Camera" ("y") w586 w620 4Pi_Capture_Actions."Setup" ("y") 4Pi_Capture_Actions."External Cycle Sync" ("y") w764 4Pi_Capture_Actions."Quit" ("y")] -> w255
            tunnel: [w258 w270 w307 w340 w364 w387 w429 w496 w535 w566 w595 w647 w664 w733 w786 TRUE] -> w253
            tunnel: FALSE -> [w258 w270 w307 w340 w364 w387 w429 w496 w535 w566 w595 w647 w664 w733 w786 _]
            tunnel: w252 -> [_ w263 w301 _ _ w372 w428 _ _ _ w583 _ _ _ _ _]
            tunnel: w251 -> [_ _ w300 _ _ w380 w425 w493 w524 _ _ _ _ _ _ _]
            tunnel: w250 -> [_ _ _ _ w363 _ _ _ _ _ _ _ _ _ _ _]
            tunnel: w249 -> [_ _ _ w339 _ _ _ _ _ _ _ _ _ _ _ _]
            tunnel: w248 -> [_ _ _ w334 _ _ _ _ _ _ _ _ _ _ _ _]
            tunnel: w247 -> [_ _ w298 _ _ w385 w426 w495 w525 _ w587 w627 w662 w732 _ _]
            tunnel: w246 -> [_ _ w295 _ _ _ w424 _ _ _ _ _ w660 w723 _ _]
            tunnel: w245 -> [w257 w269 w279 w327 w358 w375 w423 w494 w534 w564 w578 w625 w653 w717 w785 w808]
            tunnel: [w257 w269 w279 w327 w358 w375 w422 w494 w534 w564 w578 w646 w653 w717 w785 w808] -> w244
            tunnel: w243 -> [_ _ _ _ _ w368 _ _ _ _ _ _ _ _ _ _]
            tunnel: w242 -> [_ _ _ _ _ w367 _ _ _ _ _ _ _ _ _ _]
            tunnel: w241 -> [_ w268 w274 _ _ _ w421 _ _ _ w573 _ _ w721 _ _]
            frame "Idle", Default {
            }
            frame "Live Preview", "Capture" {
              w260 = FALSE ("Camera Running?")
              n255 = call "Orca Flash Messanger.vi"("Notifier Name"=w263, "Camera Actions"=Orca_Flash_Actions."STATUS") -> ("Image Ref"=w262:T5)  [unwired: 9 in, 4 out]
              n256 = Get Notifier Status(notifier=w268) -> (notifier out=w266:refnum<notifier>, current notification=w267:T6)  [unwired: 1 in, 3 out]
              n257 = Bundle By Name(cluster=w267, "Image Ref"=w262, "Cycle Number"=u16 0, "Camera Running?"=w260, "Capture?"=w260) -> (w265:T6)
              n258 = Send Notification(notification=w265, notifier=w266) -> ()  [unwired: 1 in, 2 out]
            }
            frame "Abort" {
              w278 = FALSE ("Capture?")
              w294 = u16 1 ("Current Cycle")
              w302 = FALSE ("Live Preview")
              n259 = call "Orca Flash Messanger.vi"("Notifier Name"=w301, "Camera Actions"=Orca_Flash_Actions."IDLE") -> ()  [unwired: 9 in, 5 out]
              n260 = local write "Live Preview"(w302) -> ()
              n261 = local write "Capture"(w302) -> ()
              n262 = Equal?(x=4Pi_Capture_Actions."Capture", y=w300) -> (x = y?=w280:bool)
              n263 = Get Notifier Status(notifier=w298) -> (notifier out=w305:refnum<notifier>, current notification=w304:T9)  [unwired: 1 in, 3 out]
              n264 = Bundle By Name(cluster=w304, "Running?"=FALSE) -> (w297:T9)
              n265 = local write "Current Cycle"(w294) -> ()
              n266 = local write "Current Step"(w294) -> ()
              n267 = Get Notifier Status(notifier=w274) -> (notifier out=w277:refnum<notifier>, current notification=w276:T6)  [unwired: 1 in, 3 out]
              n268 = Bundle By Name(cluster=w276, "Camera Running?"=w278, "Capture?"=w278) -> (w275:T6)
              n269 = Send Notification(notification=w297, notifier=w305) -> ()  [unwired: 1 in, 2 out]
              n270 = Unbundle By Name(w297) -> ("Metadata File Ref"=w272:refnum<file>, "Init Z Position (µm)"=w296:dbl)
              n271 = Obtain Notifier(name (unnamed)="WFDC External Sync", notification data type=T22 {"Cycle Sync"=enum."Pause Requested", "Z Offset"=0.0, "WFDC Status"=enum."Idle"} ("WFDC External Sync"), create if not found? (T)=FALSE) -> (notifier out=w290:refnum<notifier>, error out=w284:errorcluster)  [unwired: 1 in, 1 out]
              n272 = Send Notification(notification=w275, notifier=w277) -> ()  [unwired: 1 in, 2 out]
              n273 = Get Notifier Status(notifier=w290, error in (no error)=w284) -> (notifier out=w282:refnum<notifier>, current notification=w281:T22, error out=w285:errorcluster)  [unwired: 2 out]
              n274 = Unbundle By Name(w281) -> ("WFDC Status"=w289:T21)
              n275 = Unbundle By Name(w285) -> ("status"=w286:bool)
              n276 = Not A Number/Path/Refnum?(number/path/refnum=w272) -> (NaN/Path/Refnum?=w273:bool)
              n277 = case shown="True" w273 {
                tunnel: w272 -> [w309 _]
                frame False {
                  n278 = Close File(refnum=w309) -> ()  [unwired: 1 in, 2 out]
                }
                frame True {
                }
              }
              n279 = Not Equal?(x=WFDC_Status."DC Active", y=w289) -> (x != y?=w287:bool)
              n280 = Or(x=w287, y=w286) -> (x .or. y?=w283:bool)
              n281 = case shown="True" w280 {
                tunnel: w296 -> [_ w314]
                tunnel: w295 -> [_ w313]
                tunnel: w283 -> [_ w312]
                tunnel: w282 -> [_ w311]
                tunnel: w281 -> [_ w310]
                frame False {
                }
                frame True {
                  n282 = case shown="True" w312 {
                    tunnel: w314 -> [_ w326]
                    tunnel: w313 -> [_ w325]
                    tunnel: w311 -> [w319 _]
                    tunnel: w310 -> [w318 _]
                    frame False {
                      n283 = Bundle By Name(cluster=w318, "Z Offset"=0.0) -> (w320:T22)
                      n284 = Send Notification(notification=w320, notifier=w319) -> (notifier out=w315:refnum<notifier>)  [unwired: 1 in, 1 out]
                      n285 = Release Notifier(notifier=w315, force destroy? (F)=FALSE) -> ()  [unwired: 1 in, 3 out]
                    }
                    frame True {
                      n286 = Build Array(w326) -> (w321:dbl[])
                      n287 = call "Stages Messenger.vi"("Stage Notifier Name"=w325, "Actions"=Stage_Actions."MOVE", "Setpoint"=w321, "Axis"=bool[] [TRUE], "Exit While Busy?"=FALSE) -> ()  [unwired: 7 in, 4 out]
                    }
                  }
                }
              }
            }
            frame "Open Shutters", "Close Shutters" {
              n288 = Equal?(x=w338, y=4Pi_Capture_Actions."Open Shutters") -> (x = y?=w332:bool)
              n289 = Select(t=Shutter_Actions."Open" ("Action"), s=w332, f=Shutter_Actions."Close") -> (s? t:f=w333:T25)
              n290 = case shown="True" "Auto Shutter" {
                tunnel: w339 -> [_ w347]
                tunnel: w334 -> [_ w342]
                tunnel: w333 -> [_ w341]
                frame False {
                }
                frame True {
                  n291 = flat-sequence {
                    tunnel: w341 -> [w350]
                    tunnel: w347 -> [w351]
                    tunnel: [w351] -> w344
                    tunnel: [w350] -> w343
                    tunnel: w342 -> [w349]
                    tunnel: w341 -> [w348]
                    tunnel: [w354] -> w346
                    tunnel: [w353] -> w345
                    tunnel: w344 -> [w354]
                    tunnel: w343 -> [w353]
                    tunnel: w346 -> [w356]
                    tunnel: w345 -> [w355]
                    frame #0 {
                      n292 = call "Shutter Messenger.vi"("Notifier Name"=w349, "Action"=w348) -> ()  [unwired: 12 in, 2 out]
                    }
                    frame #1 {
                      n293 = Wait (ms)(milliseconds to wait=u32 100) -> ()  [unwired: 1 out]
                    }
                    frame #2 {
                      n294 = call "Shutter Messenger.vi"("Notifier Name"=w356, "Action"=w355) -> ()  [unwired: 12 in, 2 out]
                    }
                  }
                }
              }
              n295 = Select(t=4Pi_Capture_Actions."Laser On" ("y"), s=w332, f=4Pi_Capture_Actions."Laser Off") -> (s? t:f=w329:T10)
            }
            frame "Laser On", "Laser Off" {
              n296 = Equal?(x=w366, y=4Pi_Capture_Actions."Laser On") -> (x = y?=w357:bool)
              n297 = call "AOTF Messenger.vi"("AOTF Notifier Name"=w363, "AOTF Action"=AOTF_Actions."Blank", "Beam Blank"=w357) -> ()  [unwired: 7 in, 6 out]
              n298 = Select(t=4Pi_Capture_Actions."Set Exposure Time" ("y"), s=w357, f=4Pi_Capture_Actions."Quit" ("y")) -> (s? t:f=w360:T10)
            }
            frame "Set Exposure Time" {
              # "Frame Rate (Hz)"
              n299 = Get Notifier Status(notifier=w385) -> (current notification=w381:T9)  [unwired: 1 in, 4 out]
              n300 = Unbundle By Name(w381) -> ("Line Scan?"=w370:bool, "Line Scan Mode"=w369:T3, "Capture Exposure (s)"=w376:dbl, "Preview Exposure (s)"=w377:dbl)
              n301 = Equal?(x=w380, y=4Pi_Capture_Actions."Capture") -> (x = y?=w378:bool)
              n302 = Select(t=w376, s=w378, f=w377) -> (s? t:f=w374:dbl)
              n303 = case shown="True" w370 {
                tunnel: w374 -> [w389 w397]
                tunnel: [w389 w394] -> w373
                tunnel: w372 -> [w388 w396]
                tunnel: [w388 w393] -> w371
                tunnel: w369 -> [_ w392]
                tunnel: w368 -> [_ w391]
                tunnel: w367 -> [_ w390]
                frame False {
                  # "Exposure Time (s)"
                }
                frame True {
                  n304 = To Double Precision Float(number="Number of Lines") -> (double precision float=w395:dbl)
                  n305 = case shown="\"Automatic\"" w392 {
                    tunnel: w397 -> [_ w420]
                    tunnel: w396 -> [w403 w419]
                    tunnel: w395 -> [w401 w418]
                    tunnel: [w399 w417] -> w394
                    tunnel: [w402 w416] -> w393
                    tunnel: w391 -> [_ w409]
                    tunnel: w390 -> [_ w408]
                    frame Default {
                      n306 = call "Orca Flash Messanger.vi"("Notifier Name"=w403, "Camera Actions"=Orca_Flash_Actions."GETPARAM", "sCMOS Parameter"=T17 {"Value"=0.0, "Parameter"=4226016}) -> ("Notifier Name Dup"=w402:string, "sCMOS Parameter"=w406:T17)  [unwired: 8 in, 3 out]
                      n307 = Unbundle By Name(w406) -> ("Value"=w400:dbl)
                      n308 = Multiply(x=w400, y=w401) -> (x*y=w399:dbl)
                    }
                    frame "Automatic" {
                      n309 = call "4Pi Capture Set Interline Interval.vi"("Camera Notifier Name"=w419, "Frame Rate (Hz)"=w420) -> ("Camera Notifier Name (Dup)"=w416:string, "Interline Interval (s)"=w415:dbl)  [unwired: 12 in]
                      n310 = Multiply(x=w415, y=w418) -> (x*y=w417:dbl)
                      n311 = call "4Pi Capture Set Auto Waveform.vi"("Interline Interval"=w415, "Waveform Parameters"=w408) -> ("Offset (V)"=w413:dbl, "Amplitude (V)"=w412:dbl, "Samples per Channel"=w411:i32, "Delay (ms)"=w410:dbl, "Line Scan Settings"=w407:T4)  [unwired: 9 in]
                      n312 = local write "Line Scan Settings"(w407) -> ()
                      n313 = call "AO SCTR Messenger.vi"("Notifier Name"=w409, "Actions"=AO_SCTR_Actions."Update and Run", "Offset (V)"=w413, "Amplitude (V)"=w412, "Samples Per Channel"=w411, "Start Delay (ms)"=w410) -> ()  [unwired: 9 in, 1 out]
                    }
                  }
                }
              }
              n314 = Bundle By Name(cluster=T17 {"Value"=0.0, "Parameter"=2049184} ("sCMOS Parameter"), "Value"=w373) -> (w384:T17)
              n315 = call "Orca Flash Messanger.vi"("Notifier Name"=w371, "Camera Actions"=Orca_Flash_Actions."SETPARAM", "sCMOS Parameter"=w384) -> ()  [unwired: 8 in, 5 out]
            }
            frame "Start Acquisition" {
              n316 = case shown="\"Capture\"" w425 {
                tunnel: w428 -> [_ w432 _]
                tunnel: [4Pi_Capture_Actions."Quit" ("y") 4Pi_Capture_Actions."Quit" ("y") 4Pi_Capture_Actions."Update SubFolder" ("y")] -> w427
                tunnel: w426 -> [_ _ w467]
                tunnel: w424 -> [_ _ w459]
                tunnel: w423 -> [w430 w433 w455]
                tunnel: [w430 w433 w454] -> w422
                tunnel: w421 -> [_ _ w450]
                frame Default {
                }
                frame "Live Preview" {
                  n317 = call "Orca Flash Messanger.vi"("Notifier Name"=w432, "Camera Actions"=Orca_Flash_Actions."PREVIEW") -> ()  [unwired: 9 in, 5 out]
                }
                frame "Capture" {
                  w453 = sgl 0.0 ("Cycle")
                  n318 = Get Notifier Status(notifier=w450) -> (notifier out=w451:refnum<notifier>, current notification=w449:T6)  [unwired: 1 in, 3 out]
                  n319 = Bundle By Name(cluster=w449, "Capture?"=TRUE) -> (w448:T6)
                  n320 = call "Stages Messenger.vi"("Stage Notifier Name"=w459, "Actions"=Stage_Actions."Get Position") -> ("Positions"=w462:dbl[])  [unwired: 10 in, 3 out]
                  n321 = Send Notification(notification=w448, notifier=w451) -> ()  [unwired: 1 in, 2 out]
                  n322 = Index Array(array=w462, index=0) -> (element=w460:dbl)
                  n323 = local write "Z Step"(w453) -> ()
                  n324 = local write "Cycle"(w453) -> ()
                  n325 = local write "Frame"(u32 0 ("Frame")) -> ()
                  n326 = Get Notifier Status(notifier=w467) -> (notifier out=w464:refnum<notifier>, current notification=w465:T9)  [unwired: 1 in, 3 out]
                  n327 = Bundle By Name(cluster=w465, "Init Z Position (µm)"=w460) -> (w456:T9)
                  n328 = Send Notification(notification=w456, notifier=w464) -> ()  [unwired: 1 in, 2 out]
                  n329 = Unbundle By Name(w456) -> ("Cycles"=w457:u16, "No. of Z Steps"=w458:u16)
                  n330 = Bundle By Name(cluster=w455, "# of Cycles"=w457, "# of Steps"=w458) -> (w454:T20)
                  n331 = Obtain Notifier(name (unnamed)="WFDC External Sync", notification data type=T22 {"Cycle Sync"=enum."Pause Requested", "Z Offset"=0.0, "WFDC Status"=enum."Idle"} ("WFDC External Sync"), create if not found? (T)=FALSE) -> (notifier out=w437:refnum<notifier>, error out=w436:errorcluster)  [unwired: 1 in, 1 out]
                  n332 = Get Notifier Status(notifier=w437, error in (no error)=w436) -> (notifier out=w442:refnum<notifier>, current notification=w443:T22, error out=w444:errorcluster)  [unwired: 2 out]
                  n333 = Unbundle By Name(w443) -> ("WFDC Status"=w441:T21)
                  n334 = case shown="\"Error\"" w441 {
                    tunnel: w442 -> [w470 w475]
                    tunnel: w443 -> [_ w474]
                    tunnel: w444 -> [w469 w472]
                    tunnel: [w470 w473] -> w446
                    tunnel: [w469 w471] -> w445
                    frame Default {
                    }
                    frame "Error" {
                      n335 = Two Button Dialog(message="Reset Wide Field Drift Correction error?", 1:"No" ("F button name (\"Cancel\")"), 2:"Yes" ("T button name (\"OK\")")) -> (T button?=w479:bool)
                      n336 = case shown="True" w479 {
                        tunnel: w475 -> [w481 w486]
                        tunnel: w474 -> [_ w488]
                        tunnel: [w481 w484] -> w473
                        tunnel: w472 -> [w480 w483]
                        tunnel: [w480 w482] -> w471
                        frame False {
                        }
                        frame True {
                          n337 = Bundle By Name(cluster=w488, "WFDC Status"=WFDC_Status."Idle") -> (w485:T22)
                          n338 = Send Notification(notification=w485, notifier=w486, error in (no error)=w483) -> (notifier out=w484:refnum<notifier>, error out=w482:errorcluster)
                        }
                      }
                    }
                  }
                  n339 = case shown="No Error" w445 {
                    tunnel: w446 -> [w468 _]
                    frame No Error {
                      n340 = Release Notifier(notifier=w468) -> ()  [unwired: 2 in, 3 out]
                    }
                    frame Error {
                    }
                  }
                }
              }
            }
            frame "Update SubFolder" {
              n341 = Equal?(x=w493, y=4Pi_Capture_Actions."Capture") -> (x = y?=w491:bool)
              n342 = And(x=w491, y="Auto Update Subfolder") -> (x .and. y?=w489:bool)
              n343 = case shown="True" w489 {
                tunnel: w495 -> [w502 w518]
                frame False {
                  n344 = Get Notifier Status(notifier=w502) -> (notifier out=w501:refnum<notifier>, current notification=w499:T9)  [unwired: 1 in, 3 out]
                  n345 = Unbundle By Name(w499) -> ("Base Path"=w498:path)
                  n346 = Bundle By Name(cluster=w499, "Save Path"=w498) -> (w500:T9)
                  n347 = Send Notification(notification=w500, notifier=w501) -> ()  [unwired: 1 in, 2 out]
                }
                frame True {
                  n348 = Get Notifier Status(notifier=w518) -> (notifier out=w506:refnum<notifier>, current notification=w505:T9)  [unwired: 1 in, 3 out]
                  n349 = feedback #1(u32 0) -> (w508:u32)
                  n350 = Unbundle By Name(w505) -> ("Base Path"=w517:path)
                  n351 = Increment(x=w508) -> (x+1=w507:u32)
                  n352 = feedback-in #1(w507) -> ()
                  n353 = Format Into String(format string="%03d", w507) -> (resulting string=w509:string)  [unwired: 2 in, 1 out]
                  n354 = Strip Path(path=w517) -> (stripped path=w516:path, name=w514:string)
                  n355 = Concatenate Strings("Subfolder Name", w509) -> (w512:string)
                  n356 = Build Path(base path=w516, name or relative path=w512) -> (appended path=w515:path)
                  n357 = Build Path(base path=w515, name or relative path=w514) -> (appended path=w504:path)
                  n358 = Bundle By Name(cluster=w505, "Save Path"=w504) -> (w503:T9)
                  n359 = Send Notification(notification=w503, notifier=w506) -> ()  [unwired: 1 in, 2 out]
                }
              }
            }
            frame "Write Metadata" {
              n360 = Get Notifier Status(notifier=w525) -> (notifier out=w521:refnum<notifier>, current notification=w520:T9)  [unwired: 1 in, 3 out]
              n361 = Not Equal?(x=4Pi_Capture_Actions."Capture", y=w524) -> (x != y?=w526:bool)
              n362 = Unbundle By Name(w520) -> ("Init Z Position (µm)"=w519:dbl, "Save Path"=w522:path, "Z Step Size (µm)"=w530:dbl, "No. of Z Steps"=w529:u16)
              n363 = Less?(x=w529, y=u16 2) -> (x < y?=w527:bool)
              n364 = Equal To 0?(x=w530) -> (x = 0?=w528:bool)
              n365 = Compound Arithmetic op=OR(w528, w527, w526) -> (w523:bool)
              n366 = case shown="False" w523 {
                tunnel: w522 -> [w544 _]
                tunnel: w521 -> [w554 w562]
                tunnel: w520 -> [w550 w563]
                tunnel: w519 -> [w547 _]
                frame False {
                  n367 = Strip Path(path=w544) -> (stripped path=w541:path)  [unwired: 1 out]
                  n368 = call <vilib>:"Check if File or Folder Exists.vi"("path"=w541) -> ("file or folder exists?"=w543:bool, "dup path"=w542:path)  [unwired: 8 in, 1 out]
                  n369 = case shown="False" w543 {
                    tunnel: [w557 w559] -> w540
                    tunnel: w542 -> [w558 w559]
                    frame False {
                      n370 = Create Folder(path (use dialog)=w558) -> (created path=w557:path)  [unwired: 2 in, 2 out]
                    }
                    frame True {
                    }
                  }
                  n371 = Build Path(base path=w540, name or relative path="Z Positions.txt") -> (appended path=w552:path)
                  n372 = Open/Create/Replace File(file path (use dialog)=w552, operation (0:open)=T28."replace or create") -> (refnum out=w546:refnum<file>, error out=w539:errorcluster)  [unwired: 4 in, 1 out]
                  n373 = Format Value(format string="%.4f\\n", value (0)=w547) -> (output string=w545:string)  [unwired: 1 in]
                  n374 = Write to Text File(file (use dialog)=w546, text=w545, error in=w539) -> (refnum out=w537:refnum<file>, error out=w538:errorcluster)  [unwired: 1 in, 1 out]
                  n375 = case shown="Error" w538 {
                    tunnel: w537 -> [w555 _]
                    tunnel: [w555 refnum<k0> refnum] -> w536
                    frame No Error {
                    }
                    frame Error {
                    }
                  }
                  n376 = Bundle By Name(cluster=w550, "Metadata File Ref"=w536) -> (w549:T9)
                  n377 = Send Notification(notification=w549, notifier=w554) -> ()  [unwired: 1 in, 2 out]
                }
                frame True {
                  n378 = Bundle By Name(cluster=w563, "Metadata File Ref"=refnum<k0> refnum) -> (w561:T9)
                  n379 = Send Notification(notification=w561, notifier=w562) -> ()  [unwired: 1 in, 2 out]
                }
              }
            }
            frame "Setup" {
              # "Change lasers here"
            }
            frame "Camera" {
              n380 = Get Notifier Status(notifier=w587) -> (notifier out=w594:refnum<notifier>, current notification=w580:T9)  [unwired: 1 in, 3 out]
              n381 = Unbundle By Name(w578) -> ("Current Cycle"=w585:u16, "Current Step"=w584:u16)
              n382 = property on="Current Laser" class="Ring (strict)"() -> ("RingText.Text"=w579:string)  [unwired: 2 in, 2 out]
              n383 = Unbundle By Name(w580) -> ("Save Path"=w590:path, "Frames"=w581:u32)
              n384 = Get Notifier Status(notifier=w573) -> (notifier out=w577:refnum<notifier>, current notification=w576:T6)  [unwired: 1 in, 3 out]
              n385 = Bundle By Name(cluster=w576, "Camera Running?"=TRUE) -> (w574:T6)
              n386 = call "4Pi Capture File Name Increment.vi"("Step"=w584, "Cycle"=w585, "Laser Line"=w579, "Path In"=w590) -> ("Path Out"=w591:path)  [unwired: 7 in]
              n387 = call "Orca Flash Messanger.vi"("Notifier Name"=w583, "Camera Actions"=Orca_Flash_Actions."Record Settings", "Path"=w591, "# of frames"=w581) -> ("Notifier Name Dup"=w593:string)  [unwired: 7 in, 4 out]
              n388 = call "Orca Flash Messanger.vi"("Notifier Name"=w593, "Camera Actions"=Orca_Flash_Actions."RECORD") -> ("Notifier Name Dup"=w588:string, "Image Ref"=w582:T5)  [unwired: 9 in, 3 out]
              n389 = Send Notification(notification=w574, notifier=w577) -> (notifier out=w572:refnum<notifier>)  [unwired: 1 in, 1 out]
              n390 = while {
                tunnel: w588 -> [w617]
                tunnel: [w614] -> w586
                tunnel: w594 -> [w603]
                tunnel: w582 -> [w602]
                tunnel: [w596] -> w568
                tunnel: w572 -> [w596]
                stop <- w610 stop-if-true
                n391 = Get Notifier Status(notifier=w603) -> (current notification=w616:T9)  [unwired: 1 in, 4 out]
                n392 = Unbundle By Name(w616) -> ("Running?"=w609:bool)
                n393 = Wait (ms)(milliseconds to wait=u32 25) -> ()  [unwired: 1 out]
                n394 = call "IMAQ Read Custom Data"("Key"="Image Data", "Image"=w602) -> ("Custom Data Out"=w600:string)  [unwired: 7 in, 2 out]
                n395 = Unflatten From JSON(JSON string=w600, type and defaults=T29 {"Frame"=0, "Sensor Height"=0, "Sensor Width"=0, "ROI Height"=0, "ROI Width"=0, "ROI Enable?"=FALSE, "Bit per Pixel"=0} ("Camera IMAQ Key Info")) -> (value=w598:T29)  [unwired: 5 in, 1 out]
                n396 = Not(x=w609) -> (.not. x?=w613:bool)
                n397 = Unbundle By Name(w598) -> ("Frame"=→"Frame" →"Current Frame":u32)
                n398 = Select(t=Orca_Flash_Actions."STATUS" ("Camera Actions"), s=w609, f=Orca_Flash_Actions."IDLE") -> (s? t:f=w604:T19)
                n399 = call "Orca Flash Messanger.vi"("Notifier Name"=w617, "Camera Actions"=w604) -> ("Running?"=w612:bool)  [unwired: 9 in, 4 out]
                n400 = Not(x=w612) -> (.not. x?=w611:bool)
                n401 = Or(x=w613, y=w611) -> (x .or. y?=w610:bool)
                n402 = Select(t=4Pi_Capture_Actions."Switch" ("y"), s=w609, f=4Pi_Capture_Actions."Abort") -> (s? t:f=w614:T10)
              }
              n403 = Get Notifier Status(notifier=w568) -> (notifier out=w567:refnum<notifier>, current notification=w569:T6)  [unwired: 1 in, 3 out]
              n404 = Bundle By Name(cluster=w569, "Camera Running?"=FALSE) -> (w571:T6)
              n405 = Send Notification(notification=w571, notifier=w567) -> ()  [unwired: 1 in, 2 out]
            }
            frame "Switch" {
              n406 = Get Notifier Status(notifier=w627) -> (current notification=w626:T9)  [unwired: 1 in, 4 out]
              n407 = Unbundle By Name(w626) -> ("Cycles"=w622:u16, "No. of Z Steps"=w623:u16)
              n408 = Bundle By Name(cluster=w625, "# of Cycles"=w622, "# of Steps"=w623) -> (w624:T20)
              n409 = Unbundle By Name(w624) -> ("Current Cycle"=w636:u16, "# of Cycles"=w635:u16, "Current Step"=w634:u16, "# of Steps"=w633:u16)
              n410 = Increment(x=w636) -> (x+1=w619:u16)
              n411 = Increment(x=w634) -> (x+1=w618:u16)
              n412 = To Single Precision Float(number=w619) -> (single precision float=w632:sgl)
              n413 = To Single Precision Float(number=w635) -> (single precision float=w631:sgl)
              n414 = To Single Precision Float(number=w618) -> (single precision float=w630:sgl)
              n415 = To Single Precision Float(number=w633) -> (single precision float=w629:sgl)
              n416 = Divide(x=w632, y=w631) -> (x/y=→"Cycle":sgl)
              n417 = Divide(x=w630, y=w629) -> (x/y=→"Z Step":sgl)
              n418 = call "4Pi Capture Scan Counter.vi"("Scan Tracker"=w624) -> ("Scan Tracker Out"=w646:T20, "Move stage?"=w639:bool, "F_MVR/T_MOV"=w643:bool, "Exit?"=w645:bool)  [unwired: 7 in]
              n419 = Select(t=4Pi_Capture_Actions."Cycle" ("y"), s=w643, f=4Pi_Capture_Actions."Step") -> (s? t:f=w640:T10)
              n420 = Select(t=w640, s=w639, f=4Pi_Capture_Actions."Setup") -> (s? t:f=w637:T10)
              n421 = Select(t=4Pi_Capture_Actions."Abort" ("y"), s=w645, f=w637) -> (s? t:f=w620:T10)
              n422 = case shown="\"Step\"" w620 {
                tunnel: w619 -> [_ w649 _]
                tunnel: w618 -> [_ _ w651]
                frame Default {
                }
                frame "Cycle" {
                  n423 = Increment(x=w649) -> (x+1=→"Current Cycle":u16)
                }
                frame "Step" {
                  n424 = Increment(x=w651) -> (x+1=→"Current Step":u16)
                }
              }
            }
            frame "Step" {
              n425 = Get Notifier Status(notifier=w662) -> (current notification=w661:T9)  [unwired: 1 in, 4 out]
              n426 = Unbundle By Name(w661) -> ("Metadata File Ref"=w652:refnum<file>, "Z Step Size (µm)"=w654:dbl, "No. of Z Steps"=w657:u16)
              n427 = Less?(x=w657, y=u16 2) -> (x < y?=w656:bool)
              n428 = Equal To 0?(x=w654) -> (x = 0?=w659:bool)
              n429 = Or(x=w659, y=w656) -> (x .or. y?=w658:bool)
              n430 = case shown="False" w658 {
                tunnel: w660 -> [w693 _]
                tunnel: w654 -> [w692 _]
                tunnel: w653 -> [w679 _]
                tunnel: w652 -> [w669 _]
                frame False {
                  # "Force the wait to happen before the position is read."
                  n431 = Unbundle By Name(w679) -> ("Current Step"=w678:u16)
                  n432 = Obtain Notifier(name (unnamed)="WFDC External Sync", notification data type=T22 {"Cycle Sync"=enum."Pause Requested", "Z Offset"=0.0, "WFDC Status"=enum."Idle"} ("WFDC External Sync"), create if not found? (T)=FALSE) -> (notifier out=w685:refnum<notifier>, error out=w691:errorcluster)  [unwired: 1 in, 1 out]
                  n433 = Get Notifier Status(notifier=w685, error in (no error)=w691) -> (notifier out=w680:refnum<notifier>, current notification=w677:T22, error out=w690:errorcluster)  [unwired: 2 out]
                  n434 = Unbundle By Name(w677) -> ("WFDC Status"=w686:T21)
                  n435 = Unbundle By Name(w690) -> ("status"=w689:bool)
                  n436 = Not Equal?(x=WFDC_Status."DC Active", y=w686) -> (x != y?=w688:bool)
                  n437 = Or(x=w688, y=w689) -> (x .or. y?=w681:bool)
                  n438 = case shown="False" w681 {
                    tunnel: w693 -> [w698 w715]
                    tunnel: w692 -> [w705 w714]
                    tunnel: w680 -> [w702 _]
                    tunnel: w678 -> [w707 _]
                    tunnel: w677 -> [w706 _]
                    tunnel: [u32 350 ("milliseconds to wait") u32 50 ("milliseconds to wait")] -> w676
                    tunnel: [w698 w708] -> w672
                    frame False {
                      n439 = To Double Precision Float(number=w707) -> (double precision float=w704:dbl)
                      n440 = Multiply(x=w705, y=w704) -> (x*y=w703:dbl)
                      n441 = Bundle By Name(cluster=w706, "Z Offset"=w703) -> (w701:T22)
                      n442 = Send Notification(notification=w701, notifier=w702) -> (notifier out=w699:refnum<notifier>)  [unwired: 1 in, 1 out]
                      n443 = Release Notifier(notifier=w699) -> ()  [unwired: 2 in, 3 out]
                    }
                    frame True {
                      n444 = Build Array(w714) -> (w713:dbl[])
                      n445 = call "Stages Messenger.vi"("Stage Notifier Name"=w715, "Actions"=Stage_Actions."MVR", "Setpoint"=w713, "Axis"=bool[] [TRUE], "Exit While Busy?"=FALSE) -> ("Stage Notifier Name (Dup)"=w708:string)  [unwired: 7 in, 3 out]
                    }
                  }
                  n446 = Wait (ms)(milliseconds to wait=w676) -> (millisecond timer value=w665:u32)
                  n447 = Set File Position(offset (in bytes) (0)=i64 0, refnum=w669, from (0:start)=enum16{"start", "end", "current"}."end") -> (refnum out=w668:refnum<file>, error out=w666:errorcluster)  [unwired: 1 in]
                  n448 = call "Stages Messenger.vi"("Stage Notifier Name"=w672, "Actions"=Stage_Actions."Get Position", "Velocity"=w665) -> ("Positions"=w674:dbl[])  [unwired: 9 in, 3 out]
                  n449 = Index Array(array=w674, index=0) -> (element=w667:dbl)
                  n450 = case shown="No Error" w666 {
                    tunnel: w668 -> [w695 _]
                    tunnel: w667 -> [w694 _]
                    frame No Error {
                      n451 = Format Value(format string="%.4f\\n", value (0)=w694) -> (output string=w697:string)  [unwired: 1 in]
                      n452 = Write to Text File(file (use dialog)=w695, text=w697) -> ()  [unwired: 2 in, 3 out]
                    }
                    frame Error {
                    }
                  }
                }
                frame True {
                }
              }
            }
            frame "Cycle" {
              n453 = Unbundle By Name(w717) -> ("Current Cycle"=w716:u16)
              n454 = Get Notifier Status(notifier=w721) -> (notifier out=w720:refnum<notifier>, current notification=w719:T6)  [unwired: 1 in, 3 out]
              n455 = Bundle By Name(cluster=w719, "Cycle Number"=w716) -> (w718:T6)
              n456 = Get Notifier Status(notifier=w732) -> (current notification=w731:T9)  [unwired: 1 in, 4 out]
              n457 = Send Notification(notification=w718, notifier=w720) -> ()  [unwired: 1 in, 2 out]
              n458 = Unbundle By Name(w731) -> ("Init Z Position (µm)"=w722:dbl, "Z Step Size (µm)"=w727:dbl, "No. of Z Steps"=w726:u16)
              n459 = Equal To 0?(x=w727) -> (x = 0?=w730:bool)
              n460 = Less?(x=w726, y=u16 2) -> (x < y?=w729:bool)
              n461 = Or(x=w730, y=w729) -> (x .or. y?=w724:bool)
              n462 = case shown="False" w724 {
                tunnel: w723 -> [w735 _]
                tunnel: w722 -> [w737 _]
                frame False {
                  n463 = Obtain Notifier(name (unnamed)="WFDC External Sync", notification data type=T22 {"Cycle Sync"=enum."Pause Requested", "Z Offset"=0.0, "WFDC Status"=enum."Idle"} ("WFDC External Sync"), create if not found? (T)=FALSE) -> (notifier out=w743:refnum<notifier>, error out=w749:errorcluster)  [unwired: 1 in, 1 out]
                  n464 = Get Notifier Status(notifier=w743, error in (no error)=w749) -> (notifier out=w738:refnum<notifier>, current notification=w736:T22, error out=w748:errorcluster)  [unwired: 2 out]
                  n465 = Unbundle By Name(w736) -> ("WFDC Status"=w744:T21)
                  n466 = Unbundle By Name(w748) -> ("status"=w747:bool)
                  n467 = Not Equal?(x=WFDC_Status."DC Active", y=w744) -> (x != y?=w746:bool)
                  n468 = Or(x=w746, y=w747) -> (x .or. y?=w739:bool)
                  n469 = case shown="True" w739 {
                    tunnel: w738 -> [w753 _]
                    tunnel: w737 -> [_ w758]
                    tunnel: w736 -> [w752 _]
                    tunnel: w735 -> [_ w757]
                    tunnel: [u32 350 ("milliseconds to wait") u32 100 ("milliseconds to wait")] -> w734
                    frame False {
                      n470 = Bundle By Name(cluster=w752, "Z Offset"=0.0) -> (w755:T22)
                      n471 = Send Notification(notification=w755, notifier=w753) -> (notifier out=w754:refnum<notifier>)  [unwired: 1 in, 1 out]
                      n472 = Release Notifier(notifier=w754) -> ()  [unwired: 2 in, 3 out]
                    }
                    frame True {
                      n473 = Build Array(w758) -> (w759:dbl[])
                      n474 = call "Stages Messenger.vi"("Stage Notifier Name"=w757, "Actions"=Stage_Actions."MOVE", "Setpoint"=w759, "Axis"=bool[] [TRUE], "Exit While Busy?"=FALSE) -> ()  [unwired: 7 in, 4 out]
                    }
                  }
                  n475 = Wait (ms)(milliseconds to wait=w734) -> ()  [unwired: 1 out]
                }
                frame True {
                }
              }
            }
            frame "External Cycle Sync" {
              n476 = Obtain Notifier(name (unnamed)="WFDC External Sync", notification data type=T22 {"Cycle Sync"=enum."Pause Requested", "Z Offset"=0.0, "WFDC Status"=enum."Idle"} ("WFDC External Sync"), create if not found? (T)=FALSE) -> (notifier out=w781:refnum<notifier>, error out=w784:errorcluster)  [unwired: 1 in, 1 out]
              n477 = Get Notifier Status(notifier=w781, error in (no error)=w784) -> (notifier out=w770:refnum<notifier>, current notification=w769:T22, error out=w783:errorcluster)  [unwired: 2 out]
              n478 = Unbundle By Name(w783) -> ("status"=w777:bool)
              n479 = Unbundle By Name(w769) -> ("WFDC Status"=w768:T21, "Cycle Sync"=w776:T23)
              n480 = Not(x=w777) -> (.not. x?=w772:bool)
              n481 = Equal?(x=WFDC_Status."Error", y=w768) -> (x = y?=w766:bool)
              n482 = Equal?(x=WFDC_Status."DC Active", y=w768) -> (x = y?=w774:bool)
              n483 = Equal?(x=w776, y=WFDC_Cycle_Pause."Pause Requested") -> (x = y?=w773:bool)
              n484 = Compound Arithmetic op=AND(w774, w773, w772) -> (w771:bool)
              n485 = case shown="True" w771 {
                tunnel: w770 -> [_ w794]
                tunnel: w769 -> [_ w796]
                frame False {
                }
                frame True {
                  n486 = Bundle By Name(cluster=w796, "Cycle Sync"=WFDC_Cycle_Pause."Paused") -> (w793:T22)
                  n487 = Send Notification(notification=w793, notifier=w794) -> (notifier out=w792:refnum<notifier>)  [unwired: 1 in, 1 out]
                  n488 = while {
                    tunnel: w792 -> [w807]
                    tunnel: [w798] -> w789
                    tunnel: [w797] -> w791
                    i -> [w803]
                    stop <- w799 stop-if-true
                    n489 = Get Notifier Status(notifier=w807) -> (notifier out=w798:refnum<notifier>, current notification=w797:T22)  [unwired: 1 in, 3 out]
                    n490 = Greater?(x=w803, y=15000) -> (0:w800:bool)
                    n491 = Unbundle By Name(w797) -> ("Cycle Sync"=w806:T23)
                    n492 = Equal?(x=w806, y=WFDC_Cycle_Pause."Resume Requested") -> (x = y?=w801:bool)
                    n493 = Or(x=w801, y=w800) -> (x .or. y?=w799:bool)
                    n494 = Wait (ms)(milliseconds to wait=u32 1) -> ()  [unwired: 1 out]
                  }
                  n495 = Bundle By Name(cluster=w791, "Cycle Sync"=WFDC_Cycle_Pause."Resumed") -> (w788:T22)
                  n496 = Send Notification(notification=w788, notifier=w789) -> (notifier out=w787:refnum<notifier>)  [unwired: 1 in, 1 out]
                  n497 = Release Notifier(notifier=w787) -> ()  [unwired: 2 in, 3 out]
                }
              }
              n498 = Select(t=4Pi_Capture_Actions."Abort" ("y"), s=w766, f=4Pi_Capture_Actions."Setup" ("y")) -> (s? t:f=w764:T10)
            }
            frame "Quit" {
            }
          }
        }
      }
      n499 = local write "Quit"(w195) -> ()
      n500 = Release Notifier(notifier=w148) -> ()  [unwired: 2 in, 3 out]
    }
    frame Error {
      n501 = Release Notifier(notifier=w1134) -> (error out=w1133:errorcluster)  [unwired: 2 in, 2 out]
      n502 = for {
        tunnel: w1132 -> [w1139] mode=indexing
        n503 = call "IMAQ Dispose"("Image"=w1139) -> ()  [unwired: 5 in, 1 out]
      }
      n504 = Unbundle By Name(w1133) -> ("source"=w1136:string)
      n505 = Concatenate Strings("4Pi Capture Manager could not start.", "\r", w1136) -> (w1135:string)
      n506 = One Button Dialog(message=w1135) -> ()  [unwired: 1 in, 1 out]
    }
  }
  n507 = control-ref of="This VI"() -> (w96:refnum<vi>)
  n508 = property class="VI"(reference=w96) -> (reference out=w105:refnum<vi>, "Panel"=w97:refnum<vi>)  [unwired: 1 in, 1 out]
  n509 = property class="Pnl"(reference=w97) -> ("Decos[]"=w95:refnum<vi>[], "Panes[]"=w101:refnum<vi>[])  [unwired: 1 in, 2 out]
  n510 = Array Size(array=w95) -> (size(s)=w93:i32)
  n511 = Decrement(x=w93) -> (x-1=w94:i32)
  n512 = Index Array(array=w101, index=0) -> (element=w100:refnum<vi>)
  n513 = Index Array(array=w95, index=w94) -> (element=w103:refnum<vi>)
  n514 = property class="VI"(reference=w105) -> (reference out=w107:refnum<vi>, "Front Panel.PanelBounds"=w108:T31)  [unwired: 1 in, 1 out]
  n515 = property class="Decor"(reference=w103) -> ("Bounds"=w106:T32)  [unwired: 1 in, 2 out]
  n516 = property class="Pane"(reference=w100, "Origin"=T12 {"Horizontal"=0, "Vertical"=0}, "HorizScrollbarVisibility"=w104, "VertScrollbarVisibility"=w104) -> ()  [unwired: 1 in, 2 out]
  n517 = Unbundle By Name(w106) -> ("Width"=w111:u32, "Height"=w114:u32)
  n518 = control-ref of="Quit"() -> (w98:refnum<vi>)
  n519 = To Word Integer(number=w111) -> (16bit integer=w113:i16)
  n520 = To Word Integer(number=w114) -> ()  [unwired: 1 out]
  n521 = property class="Bool (strict)"(reference=w98) -> ("Height"=w116:u32, "Top"=w117:i32)  [unwired: 1 in, 2 out]
  n522 = Unbundle By Name(w108) -> ("Left"=w110:i16, "Top"=w121:i16)
  n523 = To Word Integer(number=w116) -> (16bit integer=w119:i16)
  n524 = To Word Integer(number=w117) -> (16bit integer=w120:i16)
  n525 = Add(x=w110, y=w113) -> (x+y=w112:i16)
  n526 = Compound Arithmetic op=ADD(w121, w119, w120, i16 12 ("y")) -> (w115:i16)
  n527 = Bundle By Name(cluster=w108, "Right"=w112, "Bottom"=w115) -> (w109:T31)
  n528 = property class="VI"(reference=w107, "Front Panel.PanelBounds"=w109) -> ()  [unwired: 1 in, 2 out]
